vi "GDSProject_CreateClass.vi"(0 "Project Refnum In":refnum<vi>, 1 "Project Item To Create Class Below(Use MyComputer if not wired)":refnum<vi>, 2 "ClassFolder":path=path "C:/Documents and Settings/Micke/Mina dokument/LabView/8.1 Beta/Projects/ClassFiles/MyClass3.lvclass", 3 "ClassName":string, 5 "error in (no error)":errorcluster) -> (14 "Project Refnum Out":refnum<vi>, 15 "Class Refnum Out":refnum<vi>, 16 "ClassPathOut":path, 19 "error out":errorcluster)   [LabVIEW 2020]
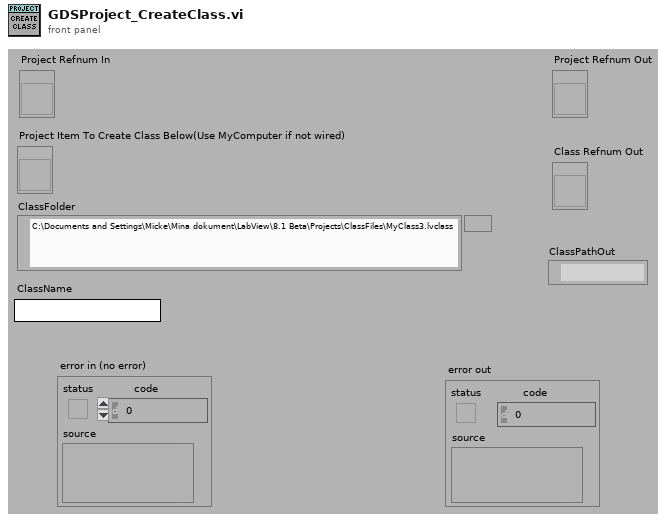
[diagram p1: front panel]
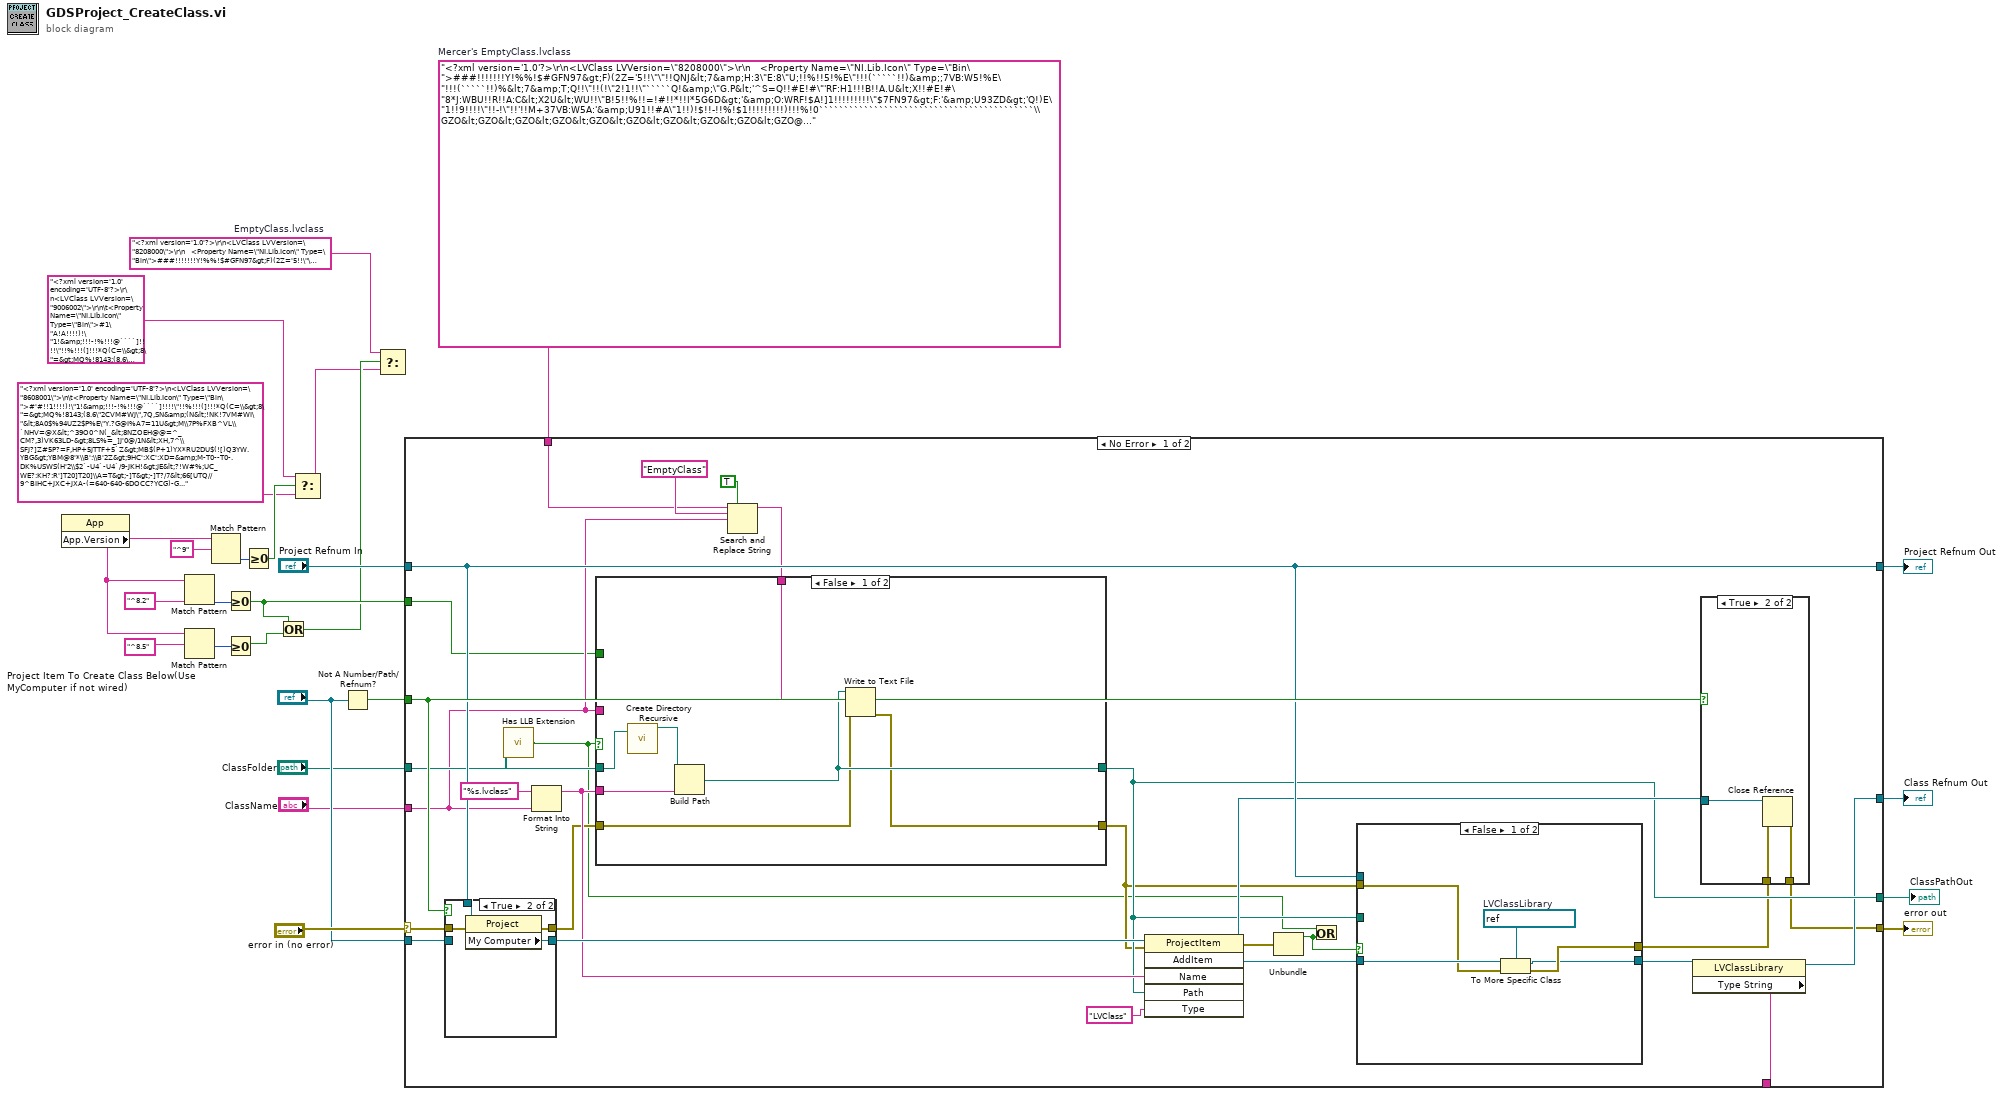
[diagram p0: block diagram]
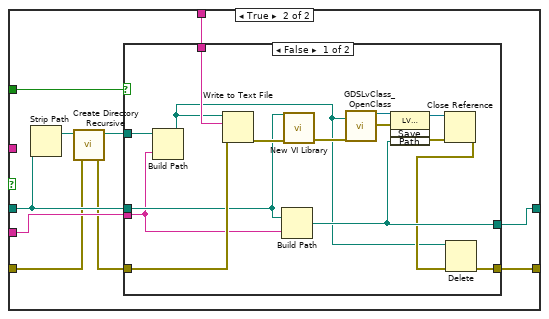
[diagram p2: hidden frame]
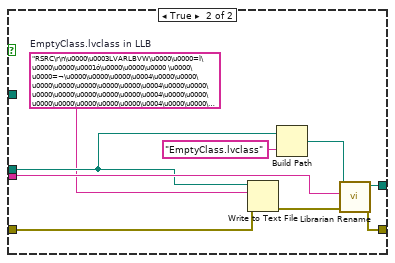
[diagram p3: hidden frame]
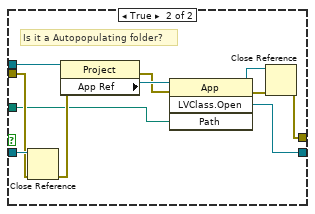
[diagram p4: hidden frame]
diagram:
  w1 = "<?xml version='1.0'?>\r\n<LVClass LVVersion=\"8208000\">\r\n   <Property Name=\"NI.Lib.Icon\" Type=\"Bin\">###!!!!!!!Y!%%!$#GFN97&gt;F)(2Z='5!!\"\"!!QNJ&lt;7&amp;H:3\"E:8\"U;!!%!!5!%E\"!!!(`````!!)&amp;;7VB:W5!%E\"!!!(`````!!)%&lt;7&amp;T;Q!!\"!!(!\"2!1!!\"`````Q!&amp;\"G.P&lt;'^S=Q!!#E!#\"'RF:H1!!!B!!A.U&lt;X!!#E!#\"8*J:WBU!!R!!A:C&lt;X2U&lt;WU!!\"B!5!!%!!=!#!!*!!I*5G6D&gt;'&amp;O:WRF!$A!]1!!!!!!!!!\"$7FN97&gt;F:'&amp;U93ZD&gt;'Q!)E\"1!!9!!!!\"!!-!\"!!'!!M+37VB:W5A:'&amp;U91!!#A\"1!!)!$!!-!!%!$1!!!!!!!!!)!!!%!0```````````````````````````````````````````\\GZO&lt;GZO&lt;GZO&lt;GZO&lt;GZO&lt;GZO&lt;GZO&lt;GZO&lt;GZO&lt;GZO@``O&lt;GZO&lt;GZO&lt;GZO&lt;GZO&lt;GZO&lt;GZO&lt;GZO&lt;GZO&lt;GZ`\\GZ``_ZO&lt;GZO&lt;GZO&lt;GZO&lt;GZO&lt;GZO&lt;GZO&lt;GZO&lt;GZO@``O&lt;H``\\GZO&lt;GZO&lt;GZO&lt;GZO&lt;GZO&lt;GZO&lt;GZO&lt;GZO&lt;GZO@_ZO@``O&lt;GZO&lt;GZO&lt;GZO&lt;GZO&lt;GZO&lt;GZO&lt;GZO&lt;GZO&lt;GZ`\\GZ``_ZO&lt;GZO&lt;GZO&lt;GZO&lt;GZO&lt;GZO&lt;GZO&lt;GZO&lt;GZO&lt;H`O&lt;H``\\GZO&lt;GZO&lt;GZO&lt;GZO&lt;GZO&lt;GZO&lt;GZO&lt;GZO&lt;GZO@_ZO@``O&lt;GZO&lt;GZO&lt;GZO&lt;GZO&lt;GZO&lt;GZO&lt;GZO&lt;GZO&lt;GZ`\\GZ``_ZO&lt;GZO&lt;GZO&lt;GZO&lt;GZO&lt;GZO&lt;GZO&lt;GZO&lt;GZO@```\\H``\\GZO&lt;GZO&lt;GZO&lt;GZO&lt;GZO&lt;GZO&lt;GZO&lt;GZO&lt;GZO&lt;GZO@```\\H`O@_Z`\\H`O@_Z`\\H`O@_Z`\\H`O@_Z`\\H`O@_Z``]!!!!!!!!!!!!!!!!!!!!!!!!!!!!!!!!!!!!!!!$``Q$``````````````Q!!!!!!!!!!!!!!!!!!!!!!!0``!0^%2%2%`U2%2%4`!!!!!!!!!!!!!!!!!!!!!!!!``]!`U2%2%4`2%2%20]!!!!!!!!!!!!!!!!!!!!!!!$``Q$`2%2%20^%2%2%`Q!!!!!!!!!!!!!!!!!!!!!!!0``!0^%2%2%`U2%2%4`!!!!!!!!!!!!!!!!!!!!!!!!``]!``````````````]!!!!!!!!!!!!!!!!!!!!!!!$``Q$`!!!!!0]!!!!!AY-!!!!!!!!!!!!!!!!!!!!!!0``!0]!!!!!`Q!!!!#$\"9/$!!!!!!!!!!!!!!!!!!!!``]!`Q!!!!$`!#-D)Y-&amp;\"17$AQ!!!!!!!!!!!!!!!!$``Q$`!!!!!0]!!!!!AQ5&amp;`Q5&amp;AY-!!!!!!!!!!!!!!0``!0````````````_$\"@```Q5&amp;\"9-D)Q!!!!!!!!!!``]!!!!!!!!!!!!!!)-&amp;\"@]&amp;\"9/$!!!!!!!!!!!!!!$``Q!!!!!!!!!!V.45AQ5&amp;\"9/$!!!!!!!!!!!!!!!!!0``!!!!!!!!!!!!!!#$\"9/$!!!!!!!!!!!!!!!!!!!!``]!!!!!!!!!!!!!!)/$!!!!!!!!!!!!!!!!!!!!!!$``Q!!!!!!!!!!!!!!!!!!!!!!!!!!!!!!!!!!!!!!!0``!!!!!!!!!!!!!!!!!!!!!!!!!!!!!!!!!!!!!!!!``]!!!!!!!!!!!!!!!!!!!!!!!!!!!!!!!!!!!!!!!$```````````````````````````````````````````]!!!#!``````````````````````````````````````````````````````````````````````````````````````````````````````````````````````````````````````````````````````````````````````````]!!!%!!0```Q$``]Q!``_:!0``:A$``T-!``]!!0`-`Q$`T-Q!`]S:!0`-:A$`T$-!`]Q!!0_:`Q$`G=Q!`ZG:!0_::A$`G4-!`ZE!!0^G`Q$`:MQ!`W;:!0^G:A$`:D-!`W9!!0]T`Q$`-]Q!`T/:!0]T:A$`-T-!`T-!!0]!`Q$`!-Q!`Q#:!0]!:A$`!$-!`Q!!!-T``Q$-`]Q!T0_:!-T`:A$-`T-!T0]!!-T-`Q$-T-Q!T-S:!-T-:A$-T$-!T-Q!!-S:`Q$-G=Q!T*G:!-S::A$-G4-!T*E!!-RG`Q$-:MQ!T';:!-RG:A$-:D-!T'9!!-QT`Q$--]Q!T$/:!-QT:A$--T-!T$-!!-Q!`Q$-!-Q!T!#:!-Q!:A$-!$-!T!!!!*H``Q#:`]Q!G@_:!*H`:A#:`T-!G@]!!*H-`Q#:T-Q!G=S:!*H-:A#:T$-!G=Q!!*G:`Q#:G=Q!G:G:!*G::A#:G4-!G:E!!*FG`Q#::MQ!G7;:!*FG:A#::D-!G79!!*ET`Q#:-]Q!G4/:!*ET:A#:-T-!G4-!!*E!`Q#:!-Q!G1#:!*E!:A#:!$-!G1!!!'&lt;``Q\"G`]Q!:P_:!'&lt;`:A\"G`T-!:P]!!'&lt;-`Q\"GT-Q!:MS:!'&lt;-:A\"GT$-!:MQ!!';:`Q\"GG=Q!:JG:!';::A\"GG4-!:JE!!':G`Q\"G:MQ!:G;:!':G:A\"G:D-!:G9!!'9T`Q\"G-]Q!:D/:!'9T:A\"G-T-!:D-!!'9!`Q\"G!-Q!:A#:!'9!:A\"G!$-!:A!!!$0``Q!T`]Q!-`_:!$0`:A!T`T-!-`]!!$0-`Q!TT-Q!-]S:!$0-:A!TT$-!-]Q!!$/:`Q!TG=Q!-ZG:!$/::A!TG4-!-ZE!!$.G`Q!T:MQ!-W;:!$.G:A!T:D-!-W9!!$-T`Q!T-]Q!-T/:!$-T:A!T-T-!-T-!!$-!`Q!T!-Q!-Q#:!$-!:A!T!$-!-Q!!!!$``Q!!`]Q!!0_:!!$`:A!!`T-!!0]!!!$-`Q!!T-Q!!-S:!!$-:A!!T$-!!-Q!!!#:`Q!!G=Q!!*G:!!#::A!!G4-!!*E!!!\"G`Q!!:MQ!!';:!!\"G:A!!:D-!!'9!!!!T`Q!!-]Q!!$/:!!!T:A!!-T-!!$-!!!!!`Q!!!-Q!!!#:!!!!:A!!!$-!\\A!!!.U!!!#\\!!!!KA!!!)A!!!\"X!!!!61!!!%1!!!!C!!!!%1!!!!$O!!!!X1!!!,M!!!#K!!!!C!!!!(=!!!\"6!!!!2!!!!#)!!!!2!!!!!/Y!!!$&gt;!!!!OQ!!!+I!!!#)!!!!&gt;Q!!!&amp;5!!!\"%!!!!)A!!!\"%!\\O\\O!.X&gt;X1#\\O\\M!KKKK!)C)C!\"X&gt;X=!6666!%2%2!!C)C)!%2%2!!!!!!!!!!!!)!!A!!!!!!!!!!%!!!#!`````Y!!!!'!!!!*A!!!'9!!!!G!!!!*A!!!#9!!!!G!!!!*A!!!(9!!!!(`````A!!!!&lt;`Y!!'TG!!\"L7A!!;VI!!'TG!!\"P`!!!;%-!!'B?Q!\"I8D!!;%*)!'`[ZY\"A!EA!9\"YQ!'!?Q!\"A!Q!!9!!!!'!!!!\"A!!!!@````]!!!#!``````````````````````````````````````````````````````````````````````````````````````````````````````````````````````````````````````````````````````````````````````````]!!!!#!0```Q!!!!!!!!!!!#!!)!!!!!!</Property>\r\n   <Property Name=\"NI.Lib.Version\" Type=\"Str\">1.0.0.0</Property>\r\n   <Property Name=\"NI.LVClass.ClassNameVisibleInProbe\" Type=\"Bool\">true</Property>\r\n   <Property Name=\"NI.LVClass.FlattenedPrivateDataCTL\" Type=\"Bin\">###!!!!!!!)!\"!!&amp;!!Q!1!!\"`````Q!!!!%!!1!!%VB35V*$$1I!!UR71U.-1F:8!!!0_!!!!W!!!!!A!!!0W!!!!\"=!!!!\"%E6N=(2Z1WRB=X-O&lt;(:D&lt;'&amp;T=Q!!!!\"Q##'!!A!Q!!!)!!!!!!!!\"!!$!$Q!P!!@1!!#!!!!!!%!!1!'`````Q!!!!!!!!!!!!!!!!!!!!!!!!!!!!!!!!!!!!!!!!!'!!!!%!!!!!!!!!!!!!!!!!!!!!!!!!!!V\"W-W9]!MA4JA!G9\\0B#@A!!!']!!5R71U-B27VQ&gt;(F$&lt;'&amp;T=SZM&gt;G.M98.T/E6N=(2Z1WRB=X-O9X2M!!!!!!!\"!!*735R#!!!!!2*&amp;&lt;8\"U?5.M98.T,GRW9WRB=X-!5&amp;2)-!!!!\"E!!1!$!!!327VQ&gt;(F$&lt;'&amp;T=SZM&gt;G.M98.T!!-!!!!!7A!!!!%!5A$RQOG`-1!!!!)327VQ&gt;(F$&lt;'&amp;T=SZM&gt;G.M98.T$E6N=(2Z1WRB=X-O9X2M!$J!5!!!(5.M&gt;8.U:8)A&lt;W9A9WRB=X-A=(*J&gt;G&amp;U:3\"E982B!!%!!!!!!!!\";!!!!\"I!#A\"D!!!\"?!!%!!1!!Q!+!'1!!!!Q!!%!#!\"A!!!!$!!+!&amp;!!!A!#!!-!#A\"D!!!!-!!\"!!B!\"Q.G&lt;'=!#%!(!W^3&gt;!!)1!=$:7^G!\"\"!5!!$!!9!\"Q!)!X6E:A!E1&amp;!!!\"V$&lt;(6T&gt;'6S)'^G)'.M98.T)(\"S;8:B&gt;'5A:'&amp;U91!+1&amp;!!!!.E:G1!#E\"1!!!$&gt;(BE!!J!5!!!!W^M:!!+1&amp;!!!!.F?(1!%A\"1!!9!#1!+!!M!$!!.!!Y!#A\"D!!!!*!!\"!!9!AQ!+!!I!9Q!!!!A!\"!!+!'-!!!!!!!1!\"!!#!!1!!1!)!'!!!!!%!$Y!5!!=!\"1!&amp;!!6!\"5!&amp;1!6!!%!!1!\"!\"5!&amp;1!6!\"5!!1!\"!!%!!1!6!\"5!&amp;1!6!\"5!&amp;1!6!\"5!&amp;A!7!\"9!#A\"E!!!!!1!8!!1!!!!+!!!1!!!%%!%!\"2!!!!]1\"!!1%!!!%2!!!\")1!!!4%!!!'$!!!\"E1!!!!!%!!!!%)?*RD9-!*'\"E9G$9!;1[9Q(]AA)IX!'E7X&amp;L*\"V!\\-.DYR&amp;!\")V#?K14)9%;)A&gt;Q,&gt;D-=M+(J!A$&amp;D2/W!!!!-!!\"6EF%5S&amp;&amp;&lt;8\"U?5.M98.T,GRW9WRB=X-[27VQ&gt;(F$&lt;'&amp;T=SZD&gt;'Q!!!!!!!!!!Q!!!*Y!!!$E?*T,9W\"AS$3W-&amp;P&amp;A!$*_3GJ)0I#%(?_W'=)IAJYDDPI#!*:!;(&gt;LAT`\"8J46$BM19J+W8?!K--4`D_9-'&amp;#@&amp;R5:(4MY1GBX4EK(-'\"17(B/RC\"MJD#X;5-/]*\"\"LNJ\\&amp;!!UQY\\]M#U3Q:)2_A,E+EA7W\"[:Q(Z:Y&amp;3).H`1-$)Q-+AT&amp;$$U-,1A_2W:X]86S1OW!]!1%1X?!!!!!!!#QAAA!!!!!-Y,D)!!!!!!)$`````A!!!!9!!!!'!!!!\"A!Q!!9!T!!'!Q-!\"AQ!Q!91!#!''!!A\"B9!Y!92A[!'%'VA\"B!;I!91&amp;7!'%\"KA\"B!69!91'K!'%\"6]\"AQ;PQ9$&amp;8Q'!.PY\"A!`Y#9!\"Y\"G!!!!*A!!!#9!!!!G!!!!*A!!!#9!!!\"W!!!!\"`````Q!!\"!$```````````````````````````````````````````]!!!!!!!!!!!!!!!!!!!!!!!!!!!!!!!!!!!!!!!$``Q!!!!!!!!!!!!!!!!!!!!!!!!!!!!!!!!!!!!!!!0``!!!!!!!!!!!!!!!!!!!!!!!!!!!!!!!!!!!!!!!!``]!!!!!!!!!!!!!!*35!!!!!!!!!!!!!!!!!!!!!!$``Q!!!!!!!!!!!*3GI+;GF!!!!!!!!!!!!!!!!!!!!0``!!!!!!!!!*3GI*K;GJKGJJ1!!!!!!!!!!!!!!!!!``]!!!!!!*3GI*K;GJK;GJK;JK;5!!!!!!!!!!!!!!$``Q!!!!#GI*K;GJK;GJK;GJK;GK;G!!!!!!!!!!!!!0``!!!!!+#AGJK;GJK;GJK;GJK;L+9!!!!!!!!!!!!!``]!!!!!I+;GI*K;GJK;GJK;L+SMI!!!!!!!!!!!!!$``Q!!!!#AJK;GJK#;GJK;L+SML+SA!!!!!!!!!!!!!0``!!!!!+#GJK;GJK;AJKSML+SML+!!!!!!!!!!!!!!``]!!!!!I+;GJK;GJK;ML+SML+SMI!!!!!!!!!!!!!$``Q!!!!#AJK;GJK;GJKSML+SML+SA!!!!!!!!!!!!!0``!!!!!+#GJK;GJK;GL+SML+SML+!!!!!!!!!!!!!!``]!!!!!I+;GJK;GJK;ML+SML+SMI!!!!!!!!!!!!!$``Q!!!!#AJK;GJK;GJKSML+SML+SA!!!!!!!!!!!!!0``!!!!!+;GJK;GJK;GL+SML+SMJK9L+SM!!!!!!!!!``]!!!!!!+#AJK;GJK;ML+SMJK;A+SML+SML!!!!!!$``Q!!!!!!!!#AJK;GJKSMJK;A+SML+SML!!!!!!!!!0``!!!!!!!!!!!!I+;GJK;;+SML+SML+Q!!!!!!!!!!``]!!!!!!!!!!!!!!+#;+SML+SML+Q!!!!!!!!$`!!$``Q!!!!!!!!!!!!!!!!!!+SML+Q!!!!!!!!!!``]!!0``!!!!!!!!!!!!!!!!!!!!!!!!!!!!!!!!!!!!`Q!!``]!!!!!!!!!!!!!!!!!!!!!!!!!!!!!!!!!!!$`!!$``Q!!!!!!!!!!!!!!!!!!!!!!!!!!!!!!!!!!!0]!!0``!!!!!!!!!!!!!!!!!!!!!!!!!!!!!!!!!!!!`Q!!``]!!!!!!!!!!!!!!!!!!!!!!!!!!!!!!!!!!!$`!!$``Q!!!!!!!!!!!!!!!!!!!!!!!!!!!!!!!!!!````!0``!!!!!!!!!!!!!!!!!!!!!!!!!!!!!!!!!!!!!!!!````````````````````````````````````````````!!!!4!!!!!%!2!$RQOG`-1!!!!)(1WRB=X-A-1N$&lt;'&amp;T=S!R,G.U&lt;!!Q1&amp;!!!\"V$&lt;(6T&gt;'6S)'^G)'.M98.T)(\"S;8:B&gt;'5A:'&amp;U91!\"!!!!!!!Q!!!!!1!E1&amp;!!!\"V$&lt;(6T&gt;'6S)'^G)'.M98.T)(\"S;8:B&gt;'5A:'&amp;U91!$!!!!!!!!!!!!-!!\"2F\")5#&amp;&amp;&lt;8\"U?5.M98.T,GRW9WRB=X-[27VQ&gt;(F$&lt;'&amp;T=SZD&gt;'Q!!!!!!!!!!Q!!!&amp;!!!!!!!!!%\"!!!!!!!&amp;A!&amp;!#-!(A!!!\"9!!!!'!!!!)Q!!!\"Y!!!!!!1!!!!!!!!!!!!!!!!!!!!!!!!!!!!!!!!!!#A!!!!!!!!!%5'&amp;O:1!!!'E!!!!!!!!%\"!!!!!!!!Q!\"!\"!!C1!!!!-!!!!#!!!!%!!!!)E!!!!!!1!!!!!!!!!!!!!!!!!!!!!!!!!!!!!!!!!!#A!!!!!!!!!&gt;1WRV=X2F=C\"P:C\"D&lt;'&amp;T=S\"Q=GFW982F)'2B&gt;'%!!!!!!!\"1!!!!!!!!\"!1!!!!!!!%!!1!/!\"I!!!!\"!!!!!A!!!!Y!!!!;!!!!!!%!!!!!!!!!!!!!!!!!!!!!!!!!!!!!!!!!!!I!!!!!!!!!\"&amp;\"B&lt;G5!!!*X!!!&amp;&amp;HC=H:1`;\".2(-&gt;`\\Z,I3T$U*5WVQ5CCP,2&amp;UM7`.@CHVN?B5AI3#QY\"/RTI&amp;IJ5H&gt;LFFB1#!3'$U,&amp;:(4)I4E8C&gt;)O41TO%TCY/&amp;O8M8@S^/^`F'CY/8MDFXLXX_8X@\\`O_\"##7:J/;!ZMW%(;%$]MW*.AC0GT:-#%?J0=_*SH)KQ#&amp;9OYU`UC%G&gt;ZD3_1X!FHCE\"_:0,%\"?!(Y2?B?]B@4,&amp;WCCWR(=QD/H[5\\&lt;&amp;5SG3S/ZOEK/]#*H!VH^(W3@'3]\"Q,%_#,:\\F/P\"F[J&amp;5]GYE!;+1O!68\"L&amp;2MOO^6A5/?+W#&gt;%F?E@^Y_(SU\"]B2XC\\SGX8-+'[VD/K\"'=.W&lt;EH@=9@Z@D^6BXVC0(Y,ROHEM^:!XC;%^Y`C&gt;N&amp;'=VGH5,R'WY9;(7$(1[(&gt;[&lt;2F45Y:0(6P'T,MQ,GQI&amp;WBBQ.SX1&amp;$@F3MZ*L)LA/F2(9H-72)S;R\"2==O'%\"[/CK\\HFQ3,PP!H3NSS))NVKN23.['P6;F8KMB=+N?&gt;^^,E.:1NCP,?!;`P@U&amp;H]YNE?9L@@*4Y\"562?U]WJ6#;Y\\Y.C78-.DSL$&lt;Y=:(B&gt;V\"L+/*A]+NK8D#S==DQS;O#-&gt;LU'\\X=9G]#[&lt;E\"6/\\%39W;OB\"N[6PP]VU.0XU21/.U\"(&gt;.SX4Q^[=!`.&amp;\\]?0`.]5-'30KDB\"GQ&lt;JL&lt;'IL23H)ZQU3_7)])EO'9Y?'0`&amp;&lt;TII\"%W+HCE35JE6ZD*F[%'J%+$2UI)XC@.E6D[(]&amp;$P3&lt;#5P.6?0$'P?!&amp;[%$Q*-\\.%&lt;H,_,E,_KW/$.R&gt;\\W,O[,7BX%%!U@%)A\"ZVP`JPOMP_I`?(Q^`GD1`OU(&amp;&amp;*P]!ITNFNQ!!!!!)!!!!)!!!\"5A!!!!Q!!&amp;#2%B1)56N=(2Z1WRB=X-O&lt;(:D&lt;'&amp;T=TJ&amp;&lt;8\"U?5.M98.T,G.U&lt;!!!!!!!!!!$!!!!@!!!!*6YH'.A9*AI)-(UD[(O,Q/4Q&amp;=A1`IP!\\/A(_.P\"A:/0Y($1*J21*,Z(Y0M8Q&lt;W8QQ-ANJA'?UDOBQ-5+$+RKBCR?2SGIG\"1Z,DM#!(7!&amp;(CQ&lt;$````69I9Q2*@DVS$KT`C!W?W8!#2+L0E7X;!O@^!*)=%!&amp;UH)5E!!!!)!!!!\"Q!!!1!!!!$`!!!!\"!!!!\"J-6E.M98.T5(*J&gt;G&amp;U:52B&gt;'&amp;597*0=G2F=AABA!)!!!!#!!1!\"Q!-!%!!!@````]!!!!\"!!%!!!!!!!!!!!!!!\"N-6E.M98.T5(*J&gt;G&amp;U:52B&gt;'&amp;5;7VF=X2B&lt;8!))9!#!!!!!1!%!!=!!1!!QOG`-1!!!!!!!!!;4&amp;:$&lt;'&amp;T=V\"S;8:B&gt;'6%982B6(FQ:52F=W-))9!#!!!!!1!)!$$`````!!%!!!!!!!Y!!!!\"!!9!5!!!!!%!!!!!!!!!!!!?4&amp;:$&lt;'&amp;T=V\"S;8:B&gt;'6%982B2':M&gt;%2B&gt;'&amp;4;8JF##'!!A!!!!%!\"!!$!!%!!!!!!!!!!!!!!!!!!!1!!!\"!!!!!+!!!!!)!!!1!!!!!!1!!!!!!!!!!!!!!!!!!!!!!!!!!!!!!!!!!!!!!!!$`!!%!!A!$!!Y!!!$I!!Y%!!!!!!Y!ZQ$7!!!!\\Q!/\"!!!!!!/!/=!VA!!!09!$A1!!!!!$A$H!.9!!!!!!!!!!!!!!!!!!!!!!!!!!!!!!!!!!!!!!!!!!!!!!!!!!!!!!!!!!!!!!!!!!!!!!!!!!!!!!!!!!!!!!!!!!!!!!!!!!!!!!!!!!!!!!!!!!!!!!!!!!!!!!!!!!!!!!!!!!!!!!!!!!!!!!!!!!!!!!!!!!!!!!!!!!!!!!!!!!!!!!!!!!!!!!!!!!!!!!!!!!!!!!!!!!!!!!!!!`1!.B!#!!!!.!.!!O1:597BP&lt;7%'6'&amp;I&lt;WVB\"F2B;'^N91%R!&amp;*45E-.#A!$4&amp;:$1UR#6F=!!!`Y!!!$9!!!!#!!!!`9!!!!!!!!!!!!!!!A!!!!.!!!!!!!!!!84%F#4A!!!!!!!!%E4&amp;:45A!!!!!!!!%Y4%FW;1!!!!!!!!&amp;-1U^/5!!!!!!!!!&amp;A6%UY-!!!!!!!!!&amp;U2%:%5Q!!!!!!!!')4%FE=Q!!!!!!!!'=6EF$2!!!!!!!!!'Q&gt;G6S=Q!!!!!!!!(%35.04A!!!!!!!!(9;7.M/!!!!!!!!!(M1V\"$-A!!!!!!!!)!2&amp;2)5!!!!!!!!!)54%FG=!!!!!!!!!)I6&amp;*F9Q!!!!)!!!)]2F\")9A!!!!!!!!*Y2F\"421!!!!!!!!+-4%FC:!!!!!!!!!+A1E2)9A!!!!!!!!+U1E2421!!!!!!!!,)6EF55Q!!!!!!!!,=466*2!!!!!!!!!,Q3%F46!!!!!!!!!-%2F2\"1A!!!!!!!!-9!!!!!0````]!!!!!!!!!!$D'MAI!!!!!`````Q!!!!!!!!!=,-;S#A!!!!$`````!!!!!!!!!*!ARL)+!!!!!0````]!!!!!!!!\"\"\"4'MAI!!!!!`````Q!!!!!!!!&amp;E#-;S#A!!!!$`````!!!!!!!!!N$]R&lt;)+!!!!!0````]!!!!!!!!$&amp;0$&amp;MAI!!!!!`````Q!!!!!!!!.)Z-7S#A!!!!4`````!!!!!!!!!_T9R&lt;)+!!!!!0````]!!!!!!!!$`-T&amp;MAI!!!!!`````Q!!!!!!!!3!Q-7S#A!!!!$`````!!!!!!!!#)3UR&lt;)+!!!!!0````]!!!!!!!!)V+D&amp;MAI!!!!!`````Q!!!!!!!!E)H-7S#A!!!!,`````!!!!!!!!#4S1R&lt;)+!!!!!`````]!!!!!!!!*E)4&amp;MAI!!!!%`````Q!!!!!!!!I!?-7S#A!!!!$`````!!!!!!!!#F2MR&lt;)+!!!!!0````]!!!!!!!!-U'$&amp;MAI!!!!!`````Q!!!!!!!!T=6-7S#A!!!!$`````!!!!!!!!$2\")R&lt;)+!!!!!0````]!!!!!!!!.E$T&amp;MAI!!!!!`````Q!!!!!!!!W=--7S#A!!!!$`````!!!!!!!!$K!ER&lt;)+!!!!!0````]!!!!!!!!/K\"D&amp;MAI!!!#!`````Q!!!!!!!!\\5$-7S#A!!!!!</Property>\r\n   <Item Name=\"EmptyClass.ctl\" Type=\"Class Private Data\" URL=\"EmptyClass.lvclass/EmptyClass.ctl\">\r\n      <Property Name=\"NI.LibItem.Scope\" Type=\"Int\">2</Property>\r\n   </Item>\r\n</LVClass>\r\n"  # Mercer's EmptyClass.lvclass
  w9 = "<?xml version='1.0'?>\r\n<LVClass LVVersion=\"8208000\">\r\n   <Property Name=\"NI.Lib.Icon\" Type=\"Bin\">###!!!!!!!Y!%%!$#GFN97&gt;F)(2Z='5!!\"\"!!QNJ&lt;7&amp;H:3\"E:8\"U;!!%!!5!%E\"!!!(`````!!)&amp;;7VB:W5!%E\"!!!(`````!!)%&lt;7&amp;T;Q!!\"!!(!\"2!1!!\"`````Q!&amp;\"G.P&lt;'^S=Q!!#E!#\"'RF:H1!!!B!!A.U&lt;X!!#E!#\"8*J:WBU!!R!!A:C&lt;X2U&lt;WU!!\"B!5!!%!!=!#!!*!!I*5G6D&gt;'&amp;O:WRF!$A!]1!!!!!!!!!\"$7FN97&gt;F:'&amp;U93ZD&gt;'Q!)E\"1!!9!!!!\"!!-!\"!!'!!M+37VB:W5A:'&amp;U91!!#A\"1!!)!$!!-!!%!$1!!!!!!!!!)!!!%!0```````````````````````````````````````````\\GZO&lt;GZO&lt;GZO&lt;GZO&lt;GZO&lt;GZO&lt;GZO&lt;GZO&lt;GZO&lt;GZO@``O&lt;GZO&lt;GZO&lt;GZO&lt;GZO&lt;GZO&lt;GZO&lt;GZO&lt;GZO&lt;GZ`\\GZ``_ZO&lt;GZO&lt;GZO&lt;GZO&lt;GZO&lt;GZO&lt;GZO&lt;GZO&lt;GZO@``O&lt;H``\\GZO&lt;GZO&lt;GZO&lt;GZO&lt;GZO&lt;GZO&lt;GZO&lt;GZO&lt;GZO@_ZO@``O&lt;GZO&lt;GZO&lt;GZO&lt;GZO&lt;GZO&lt;GZO&lt;GZO&lt;GZO&lt;GZ`\\GZ``_ZO&lt;GZO&lt;GZO&lt;GZO&lt;GZO&lt;GZO&lt;GZO&lt;GZO&lt;GZO&lt;H`O&lt;H``\\GZO&lt;GZO&lt;GZO&lt;GZO&lt;GZO&lt;GZO&lt;GZO&lt;GZO&lt;GZO@_ZO@``O&lt;GZO&lt;GZO&lt;GZO&lt;GZO&lt;GZO&lt;GZO&lt;GZO&lt;GZO&lt;GZ`\\GZ``_ZO&lt;GZO&lt;GZO&lt;GZO&lt;GZO&lt;GZO&lt;GZO&lt;GZO&lt;GZO@```\\H``\\GZO&lt;GZO&lt;GZO&lt;GZO&lt;GZO&lt;GZO&lt;GZO&lt;GZO&lt;GZO&lt;GZO@```\\H`O@_Z`\\H`O@_Z`\\H`O@_Z`\\H`O@_Z`\\H`O@_Z``]!!!!!!!!!!!!!!!!!!!!!!!!!!!!!!!!!!!!!!!$``Q$``````````````Q!!!!!!!!!!!!!!!!!!!!!!!0``!0^%2%2%`U2%2%4`!!!!!!!!!!!!!!!!!!!!!!!!``]!`U2%2%4`2%2%20]!!!!!!!!!!!!!!!!!!!!!!!$``Q$`2%2%20^%2%2%`Q!!!!!!!!!!!!!!!!!!!!!!!0``!0^%2%2%`U2%2%4`!!!!!!!!!!!!!!!!!!!!!!!!``]!``````````````]!!!!!!!!!!!!!!!!!!!!!!!$``Q$`!!!!!0]!!!!!AY-!!!!!!!!!!!!!!!!!!!!!!0``!0]!!!!!`Q!!!!#$\"9/$!!!!!!!!!!!!!!!!!!!!``]!`Q!!!!$`!#-D)Y-&amp;\"17$AQ!!!!!!!!!!!!!!!!$``Q$`!!!!!0]!!!!!AQ5&amp;`Q5&amp;AY-!!!!!!!!!!!!!!0``!0````````````_$\"@```Q5&amp;\"9-D)Q!!!!!!!!!!``]!!!!!!!!!!!!!!)-&amp;\"@]&amp;\"9/$!!!!!!!!!!!!!!$``Q!!!!!!!!!!V.45AQ5&amp;\"9/$!!!!!!!!!!!!!!!!!0``!!!!!!!!!!!!!!#$\"9/$!!!!!!!!!!!!!!!!!!!!``]!!!!!!!!!!!!!!)/$!!!!!!!!!!!!!!!!!!!!!!$``Q!!!!!!!!!!!!!!!!!!!!!!!!!!!!!!!!!!!!!!!0``!!!!!!!!!!!!!!!!!!!!!!!!!!!!!!!!!!!!!!!!``]!!!!!!!!!!!!!!!!!!!!!!!!!!!!!!!!!!!!!!!$```````````````````````````````````````````]!!!#!``````````````````````````````````````````````````````````````````````````````````````````````````````````````````````````````````````````````````````````````````````````]!!!%!!0```Q$``]Q!``_:!0``:A$``T-!``]!!0`-`Q$`T-Q!`]S:!0`-:A$`T$-!`]Q!!0_:`Q$`G=Q!`ZG:!0_::A$`G4-!`ZE!!0^G`Q$`:MQ!`W;:!0^G:A$`:D-!`W9!!0]T`Q$`-]Q!`T/:!0]T:A$`-T-!`T-!!0]!`Q$`!-Q!`Q#:!0]!:A$`!$-!`Q!!!-T``Q$-`]Q!T0_:!-T`:A$-`T-!T0]!!-T-`Q$-T-Q!T-S:!-T-:A$-T$-!T-Q!!-S:`Q$-G=Q!T*G:!-S::A$-G4-!T*E!!-RG`Q$-:MQ!T';:!-RG:A$-:D-!T'9!!-QT`Q$--]Q!T$/:!-QT:A$--T-!T$-!!-Q!`Q$-!-Q!T!#:!-Q!:A$-!$-!T!!!!*H``Q#:`]Q!G@_:!*H`:A#:`T-!G@]!!*H-`Q#:T-Q!G=S:!*H-:A#:T$-!G=Q!!*G:`Q#:G=Q!G:G:!*G::A#:G4-!G:E!!*FG`Q#::MQ!G7;:!*FG:A#::D-!G79!!*ET`Q#:-]Q!G4/:!*ET:A#:-T-!G4-!!*E!`Q#:!-Q!G1#:!*E!:A#:!$-!G1!!!'&lt;``Q\"G`]Q!:P_:!'&lt;`:A\"G`T-!:P]!!'&lt;-`Q\"GT-Q!:MS:!'&lt;-:A\"GT$-!:MQ!!';:`Q\"GG=Q!:JG:!';::A\"GG4-!:JE!!':G`Q\"G:MQ!:G;:!':G:A\"G:D-!:G9!!'9T`Q\"G-]Q!:D/:!'9T:A\"G-T-!:D-!!'9!`Q\"G!-Q!:A#:!'9!:A\"G!$-!:A!!!$0``Q!T`]Q!-`_:!$0`:A!T`T-!-`]!!$0-`Q!TT-Q!-]S:!$0-:A!TT$-!-]Q!!$/:`Q!TG=Q!-ZG:!$/::A!TG4-!-ZE!!$.G`Q!T:MQ!-W;:!$.G:A!T:D-!-W9!!$-T`Q!T-]Q!-T/:!$-T:A!T-T-!-T-!!$-!`Q!T!-Q!-Q#:!$-!:A!T!$-!-Q!!!!$``Q!!`]Q!!0_:!!$`:A!!`T-!!0]!!!$-`Q!!T-Q!!-S:!!$-:A!!T$-!!-Q!!!#:`Q!!G=Q!!*G:!!#::A!!G4-!!*E!!!\"G`Q!!:MQ!!';:!!\"G:A!!:D-!!'9!!!!T`Q!!-]Q!!$/:!!!T:A!!-T-!!$-!!!!!`Q!!!-Q!!!#:!!!!:A!!!$-!\\A!!!.U!!!#\\!!!!KA!!!)A!!!\"X!!!!61!!!%1!!!!C!!!!%1!!!!$O!!!!X1!!!,M!!!#K!!!!C!!!!(=!!!\"6!!!!2!!!!#)!!!!2!!!!!/Y!!!$&gt;!!!!OQ!!!+I!!!#)!!!!&gt;Q!!!&amp;5!!!\"%!!!!)A!!!\"%!\\O\\O!.X&gt;X1#\\O\\M!KKKK!)C)C!\"X&gt;X=!6666!%2%2!!C)C)!%2%2!!!!!!!!!!!!)!!A!!!!!!!!!!%!!!#!`````Y!!!!'!!!!*A!!!'9!!!!G!!!!*A!!!#9!!!!G!!!!*A!!!(9!!!!(`````A!!!!&lt;`Y!!'TG!!\"L7A!!;VI!!'TG!!\"P`!!!;%-!!'B?Q!\"I8D!!;%*)!'`[ZY\"A!EA!9\"YQ!'!?Q!\"A!Q!!9!!!!'!!!!\"A!!!!@````]!!!#!``````````````````````````````````````````````````````````````````````````````````````````````````````````````````````````````````````````````````````````````````````````]!!!!#!0```Q!!!!!!!!!!!#!!)!!!!!!</Property>\r\n   <Property Name=\"NI.Lib.Version\" Type=\"Str\">1.0.0.0</Property>\r\n   <Property Name=\"NI.LVClass.ClassNameVisibleInProbe\" Type=\"Bool\">true</Property>\r\n   <Property Name=\"NI.LVClass.FlattenedPrivateDataCTL\" Type=\"Bin\">###!!!!!!!)!\"!!&amp;!!Q!1!!\"`````Q!!!!%!!1!!%VB35V*$$1I!!UR71U.-1F:8!!!0_!!!!W!!!!!A!!!0W!!!!\"=!!!!\"%E6N=(2Z1WRB=X-O&lt;(:D&lt;'&amp;T=Q!!!!\"Q##'!!A!Q!!!)!!!!!!!!\"!!$!$Q!P!!@1!!#!!!!!!%!!1!'`````Q!!!!!!!!!!!!!!!!!!!!!!!!!!!!!!!!!!!!!!!!!'!!!!%!!!!!!!!!!!!!!!!!!!!!!!!!!!V\"W-W9]!MA4JA!G9\\0B#@A!!!']!!5R71U-B27VQ&gt;(F$&lt;'&amp;T=SZM&gt;G.M98.T/E6N=(2Z1WRB=X-O9X2M!!!!!!!\"!!*735R#!!!!!2*&amp;&lt;8\"U?5.M98.T,GRW9WRB=X-!5&amp;2)-!!!!\"E!!1!$!!!327VQ&gt;(F$&lt;'&amp;T=SZM&gt;G.M98.T!!-!!!!!7A!!!!%!5A$RQOG`-1!!!!)327VQ&gt;(F$&lt;'&amp;T=SZM&gt;G.M98.T$E6N=(2Z1WRB=X-O9X2M!$J!5!!!(5.M&gt;8.U:8)A&lt;W9A9WRB=X-A=(*J&gt;G&amp;U:3\"E982B!!%!!!!!!!!\";!!!!\"I!#A\"D!!!\"?!!%!!1!!Q!+!'1!!!!Q!!%!#!\"A!!!!$!!+!&amp;!!!A!#!!-!#A\"D!!!!-!!\"!!B!\"Q.G&lt;'=!#%!(!W^3&gt;!!)1!=$:7^G!\"\"!5!!$!!9!\"Q!)!X6E:A!E1&amp;!!!\"V$&lt;(6T&gt;'6S)'^G)'.M98.T)(\"S;8:B&gt;'5A:'&amp;U91!+1&amp;!!!!.E:G1!#E\"1!!!$&gt;(BE!!J!5!!!!W^M:!!+1&amp;!!!!.F?(1!%A\"1!!9!#1!+!!M!$!!.!!Y!#A\"D!!!!*!!\"!!9!AQ!+!!I!9Q!!!!A!\"!!+!'-!!!!!!!1!\"!!#!!1!!1!)!'!!!!!%!$Y!5!!=!\"1!&amp;!!6!\"5!&amp;1!6!!%!!1!\"!\"5!&amp;1!6!\"5!!1!\"!!%!!1!6!\"5!&amp;1!6!\"5!&amp;1!6!\"5!&amp;A!7!\"9!#A\"E!!!!!1!8!!1!!!!+!!!1!!!%%!%!\"2!!!!]1\"!!1%!!!%2!!!\")1!!!4%!!!'$!!!\"E1!!!!!%!!!!%)?*RD9-!*'\"E9G$9!;1[9Q(]AA)IX!'E7X&amp;L*\"V!\\-.DYR&amp;!\")V#?K14)9%;)A&gt;Q,&gt;D-=M+(J!A$&amp;D2/W!!!!-!!\"6EF%5S&amp;&amp;&lt;8\"U?5.M98.T,GRW9WRB=X-[27VQ&gt;(F$&lt;'&amp;T=SZD&gt;'Q!!!!!!!!!!Q!!!*Y!!!$E?*T,9W\"AS$3W-&amp;P&amp;A!$*_3GJ)0I#%(?_W'=)IAJYDDPI#!*:!;(&gt;LAT`\"8J46$BM19J+W8?!K--4`D_9-'&amp;#@&amp;R5:(4MY1GBX4EK(-'\"17(B/RC\"MJD#X;5-/]*\"\"LNJ\\&amp;!!UQY\\]M#U3Q:)2_A,E+EA7W\"[:Q(Z:Y&amp;3).H`1-$)Q-+AT&amp;$$U-,1A_2W:X]86S1OW!]!1%1X?!!!!!!!#QAAA!!!!!-Y,D)!!!!!!)$`````A!!!!9!!!!'!!!!\"A!Q!!9!T!!'!Q-!\"AQ!Q!91!#!''!!A\"B9!Y!92A[!'%'VA\"B!;I!91&amp;7!'%\"KA\"B!69!91'K!'%\"6]\"AQ;PQ9$&amp;8Q'!.PY\"A!`Y#9!\"Y\"G!!!!*A!!!#9!!!!G!!!!*A!!!#9!!!\"W!!!!\"`````Q!!\"!$```````````````````````````````````````````]!!!!!!!!!!!!!!!!!!!!!!!!!!!!!!!!!!!!!!!$``Q!!!!!!!!!!!!!!!!!!!!!!!!!!!!!!!!!!!!!!!0``!!!!!!!!!!!!!!!!!!!!!!!!!!!!!!!!!!!!!!!!``]!!!!!!!!!!!!!!*35!!!!!!!!!!!!!!!!!!!!!!$``Q!!!!!!!!!!!*3GI+;GF!!!!!!!!!!!!!!!!!!!!0``!!!!!!!!!*3GI*K;GJKGJJ1!!!!!!!!!!!!!!!!!``]!!!!!!*3GI*K;GJK;GJK;JK;5!!!!!!!!!!!!!!$``Q!!!!#GI*K;GJK;GJK;GJK;GK;G!!!!!!!!!!!!!0``!!!!!+#AGJK;GJK;GJK;GJK;L+9!!!!!!!!!!!!!``]!!!!!I+;GI*K;GJK;GJK;L+SMI!!!!!!!!!!!!!$``Q!!!!#AJK;GJK#;GJK;L+SML+SA!!!!!!!!!!!!!0``!!!!!+#GJK;GJK;AJKSML+SML+!!!!!!!!!!!!!!``]!!!!!I+;GJK;GJK;ML+SML+SMI!!!!!!!!!!!!!$``Q!!!!#AJK;GJK;GJKSML+SML+SA!!!!!!!!!!!!!0``!!!!!+#GJK;GJK;GL+SML+SML+!!!!!!!!!!!!!!``]!!!!!I+;GJK;GJK;ML+SML+SMI!!!!!!!!!!!!!$``Q!!!!#AJK;GJK;GJKSML+SML+SA!!!!!!!!!!!!!0``!!!!!+;GJK;GJK;GL+SML+SMJK9L+SM!!!!!!!!!``]!!!!!!+#AJK;GJK;ML+SMJK;A+SML+SML!!!!!!$``Q!!!!!!!!#AJK;GJKSMJK;A+SML+SML!!!!!!!!!0``!!!!!!!!!!!!I+;GJK;;+SML+SML+Q!!!!!!!!!!``]!!!!!!!!!!!!!!+#;+SML+SML+Q!!!!!!!!$`!!$``Q!!!!!!!!!!!!!!!!!!+SML+Q!!!!!!!!!!``]!!0``!!!!!!!!!!!!!!!!!!!!!!!!!!!!!!!!!!!!`Q!!``]!!!!!!!!!!!!!!!!!!!!!!!!!!!!!!!!!!!$`!!$``Q!!!!!!!!!!!!!!!!!!!!!!!!!!!!!!!!!!!0]!!0``!!!!!!!!!!!!!!!!!!!!!!!!!!!!!!!!!!!!`Q!!``]!!!!!!!!!!!!!!!!!!!!!!!!!!!!!!!!!!!$`!!$``Q!!!!!!!!!!!!!!!!!!!!!!!!!!!!!!!!!!````!0``!!!!!!!!!!!!!!!!!!!!!!!!!!!!!!!!!!!!!!!!````````````````````````````````````````````!!!!4!!!!!%!2!$RQOG`-1!!!!)(1WRB=X-A-1N$&lt;'&amp;T=S!R,G.U&lt;!!Q1&amp;!!!\"V$&lt;(6T&gt;'6S)'^G)'.M98.T)(\"S;8:B&gt;'5A:'&amp;U91!\"!!!!!!!Q!!!!!1!E1&amp;!!!\"V$&lt;(6T&gt;'6S)'^G)'.M98.T)(\"S;8:B&gt;'5A:'&amp;U91!$!!!!!!!!!!!!-!!\"2F\")5#&amp;&amp;&lt;8\"U?5.M98.T,GRW9WRB=X-[27VQ&gt;(F$&lt;'&amp;T=SZD&gt;'Q!!!!!!!!!!Q!!!&amp;!!!!!!!!!%\"!!!!!!!&amp;A!&amp;!#-!(A!!!\"9!!!!'!!!!)Q!!!\"Y!!!!!!1!!!!!!!!!!!!!!!!!!!!!!!!!!!!!!!!!!#A!!!!!!!!!%5'&amp;O:1!!!'E!!!!!!!!%\"!!!!!!!!Q!\"!\"!!C1!!!!-!!!!#!!!!%!!!!)E!!!!!!1!!!!!!!!!!!!!!!!!!!!!!!!!!!!!!!!!!#A!!!!!!!!!&gt;1WRV=X2F=C\"P:C\"D&lt;'&amp;T=S\"Q=GFW982F)'2B&gt;'%!!!!!!!\"1!!!!!!!!\"!1!!!!!!!%!!1!/!\"I!!!!\"!!!!!A!!!!Y!!!!;!!!!!!%!!!!!!!!!!!!!!!!!!!!!!!!!!!!!!!!!!!I!!!!!!!!!\"&amp;\"B&lt;G5!!!*X!!!&amp;&amp;HC=H:1`;\".2(-&gt;`\\Z,I3T$U*5WVQ5CCP,2&amp;UM7`.@CHVN?B5AI3#QY\"/RTI&amp;IJ5H&gt;LFFB1#!3'$U,&amp;:(4)I4E8C&gt;)O41TO%TCY/&amp;O8M8@S^/^`F'CY/8MDFXLXX_8X@\\`O_\"##7:J/;!ZMW%(;%$]MW*.AC0GT:-#%?J0=_*SH)KQ#&amp;9OYU`UC%G&gt;ZD3_1X!FHCE\"_:0,%\"?!(Y2?B?]B@4,&amp;WCCWR(=QD/H[5\\&lt;&amp;5SG3S/ZOEK/]#*H!VH^(W3@'3]\"Q,%_#,:\\F/P\"F[J&amp;5]GYE!;+1O!68\"L&amp;2MOO^6A5/?+W#&gt;%F?E@^Y_(SU\"]B2XC\\SGX8-+'[VD/K\"'=.W&lt;EH@=9@Z@D^6BXVC0(Y,ROHEM^:!XC;%^Y`C&gt;N&amp;'=VGH5,R'WY9;(7$(1[(&gt;[&lt;2F45Y:0(6P'T,MQ,GQI&amp;WBBQ.SX1&amp;$@F3MZ*L)LA/F2(9H-72)S;R\"2==O'%\"[/CK\\HFQ3,PP!H3NSS))NVKN23.['P6;F8KMB=+N?&gt;^^,E.:1NCP,?!;`P@U&amp;H]YNE?9L@@*4Y\"562?U]WJ6#;Y\\Y.C78-.DSL$&lt;Y=:(B&gt;V\"L+/*A]+NK8D#S==DQS;O#-&gt;LU'\\X=9G]#[&lt;E\"6/\\%39W;OB\"N[6PP]VU.0XU21/.U\"(&gt;.SX4Q^[=!`.&amp;\\]?0`.]5-'30KDB\"GQ&lt;JL&lt;'IL23H)ZQU3_7)])EO'9Y?'0`&amp;&lt;TII\"%W+HCE35JE6ZD*F[%'J%+$2UI)XC@.E6D[(]&amp;$P3&lt;#5P.6?0$'P?!&amp;[%$Q*-\\.%&lt;H,_,E,_KW/$.R&gt;\\W,O[,7BX%%!U@%)A\"ZVP`JPOMP_I`?(Q^`GD1`OU(&amp;&amp;*P]!ITNFNQ!!!!!)!!!!)!!!\"5A!!!!Q!!&amp;#2%B1)56N=(2Z1WRB=X-O&lt;(:D&lt;'&amp;T=TJ&amp;&lt;8\"U?5.M98.T,G.U&lt;!!!!!!!!!!$!!!!@!!!!*6YH'.A9*AI)-(UD[(O,Q/4Q&amp;=A1`IP!\\/A(_.P\"A:/0Y($1*J21*,Z(Y0M8Q&lt;W8QQ-ANJA'?UDOBQ-5+$+RKBCR?2SGIG\"1Z,DM#!(7!&amp;(CQ&lt;$````69I9Q2*@DVS$KT`C!W?W8!#2+L0E7X;!O@^!*)=%!&amp;UH)5E!!!!)!!!!\"Q!!!1!!!!$`!!!!\"!!!!\"J-6E.M98.T5(*J&gt;G&amp;U:52B&gt;'&amp;597*0=G2F=AABA!)!!!!#!!1!\"Q!-!%!!!@````]!!!!\"!!%!!!!!!!!!!!!!!\"N-6E.M98.T5(*J&gt;G&amp;U:52B&gt;'&amp;5;7VF=X2B&lt;8!))9!#!!!!!1!%!!=!!1!!QOG`-1!!!!!!!!!;4&amp;:$&lt;'&amp;T=V\"S;8:B&gt;'6%982B6(FQ:52F=W-))9!#!!!!!1!)!$$`````!!%!!!!!!!Y!!!!\"!!9!5!!!!!%!!!!!!!!!!!!?4&amp;:$&lt;'&amp;T=V\"S;8:B&gt;'6%982B2':M&gt;%2B&gt;'&amp;4;8JF##'!!A!!!!%!\"!!$!!%!!!!!!!!!!!!!!!!!!!1!!!\"!!!!!+!!!!!)!!!1!!!!!!1!!!!!!!!!!!!!!!!!!!!!!!!!!!!!!!!!!!!!!!!$`!!%!!A!$!!Y!!!$I!!Y%!!!!!!Y!ZQ$7!!!!\\Q!/\"!!!!!!/!/=!VA!!!09!$A1!!!!!$A$H!.9!!!!!!!!!!!!!!!!!!!!!!!!!!!!!!!!!!!!!!!!!!!!!!!!!!!!!!!!!!!!!!!!!!!!!!!!!!!!!!!!!!!!!!!!!!!!!!!!!!!!!!!!!!!!!!!!!!!!!!!!!!!!!!!!!!!!!!!!!!!!!!!!!!!!!!!!!!!!!!!!!!!!!!!!!!!!!!!!!!!!!!!!!!!!!!!!!!!!!!!!!!!!!!!!!!!!!!!!!`1!.B!#!!!!.!.!!O1:597BP&lt;7%'6'&amp;I&lt;WVB\"F2B;'^N91%R!&amp;*45E-.#A!$4&amp;:$1UR#6F=!!!`Y!!!$9!!!!#!!!!`9!!!!!!!!!!!!!!!A!!!!.!!!!!!!!!!84%F#4A!!!!!!!!%E4&amp;:45A!!!!!!!!%Y4%FW;1!!!!!!!!&amp;-1U^/5!!!!!!!!!&amp;A6%UY-!!!!!!!!!&amp;U2%:%5Q!!!!!!!!')4%FE=Q!!!!!!!!'=6EF$2!!!!!!!!!'Q&gt;G6S=Q!!!!!!!!(%35.04A!!!!!!!!(9;7.M/!!!!!!!!!(M1V\"$-A!!!!!!!!)!2&amp;2)5!!!!!!!!!)54%FG=!!!!!!!!!)I6&amp;*F9Q!!!!)!!!)]2F\")9A!!!!!!!!*Y2F\"421!!!!!!!!+-4%FC:!!!!!!!!!+A1E2)9A!!!!!!!!+U1E2421!!!!!!!!,)6EF55Q!!!!!!!!,=466*2!!!!!!!!!,Q3%F46!!!!!!!!!-%2F2\"1A!!!!!!!!-9!!!!!0````]!!!!!!!!!!$D'MAI!!!!!`````Q!!!!!!!!!=,-;S#A!!!!$`````!!!!!!!!!*!ARL)+!!!!!0````]!!!!!!!!\"\"\"4'MAI!!!!!`````Q!!!!!!!!&amp;E#-;S#A!!!!$`````!!!!!!!!!N$]R&lt;)+!!!!!0````]!!!!!!!!$&amp;0$&amp;MAI!!!!!`````Q!!!!!!!!.)Z-7S#A!!!!4`````!!!!!!!!!_T9R&lt;)+!!!!!0````]!!!!!!!!$`-T&amp;MAI!!!!!`````Q!!!!!!!!3!Q-7S#A!!!!$`````!!!!!!!!#)3UR&lt;)+!!!!!0````]!!!!!!!!)V+D&amp;MAI!!!!!`````Q!!!!!!!!E)H-7S#A!!!!,`````!!!!!!!!#4S1R&lt;)+!!!!!`````]!!!!!!!!*E)4&amp;MAI!!!!%`````Q!!!!!!!!I!?-7S#A!!!!$`````!!!!!!!!#F2MR&lt;)+!!!!!0````]!!!!!!!!-U'$&amp;MAI!!!!!`````Q!!!!!!!!T=6-7S#A!!!!$`````!!!!!!!!$2\")R&lt;)+!!!!!0````]!!!!!!!!.E$T&amp;MAI!!!!!`````Q!!!!!!!!W=--7S#A!!!!$`````!!!!!!!!$K!ER&lt;)+!!!!!0````]!!!!!!!!/K\"D&amp;MAI!!!#!`````Q!!!!!!!!\\5$-7S#A!!!!!</Property>\r\n   <Property Name=\"NI.LVClass.Geneology\" Type=\"Xml\"><String>\r\r\n<Name></Name>\r\r\n<Val>!!!!!1!!!!%327VQ&gt;(F$&lt;'&amp;T=SZM&gt;G.M98.T!&amp;\"53$!!!!!!!!!!!!!!!!%!!1!!!!!!!!!!!!%!\"A\"1!!!!!1!!!!!!!!!!!!!!!1Z-97*73568)%^C;G6D&gt;!\"16%AQ!!!!!!!!!!!!##'!!A!!!!!</Val>\r\r\n</String>\r\r\n</Property>\r\n   <Item Name=\"EmptyClass.ctl\" Type=\"Class Private Data\" URL=\"EmptyClass.lvclass/EmptyClass.ctl\">\r\n      <Property Name=\"NI.LibItem.Scope\" Type=\"Int\">2</Property>\r\n   </Item>\r\n</LVClass>\r\n"  # EmptyClass.lvclass
  n1 = property class="App"() -> ("App.Version"=w7:string)  [unwired: 2 in, 2 out]
  n2 = Match Pattern(string=w7, regular expression="^8.2") -> (offset past match=w16:i32)  [unwired: 1 in, 3 out]
  n3 = Match Pattern(string=w7, regular expression="^8.5") -> (offset past match=w13:i32)  [unwired: 1 in, 3 out]
  n4 = Match Pattern(string=w7, regular expression="^9") -> (offset past match=w6:i32)  [unwired: 1 in, 3 out]
  n5 = Greater Or Equal To 0?(x=w16) -> (x >= 0?=w12:bool)
  n6 = Greater Or Equal To 0?(x=w13) -> (x >= 0?=w11:bool)
  n7 = Greater Or Equal To 0?(x=w6) -> (x >= 0?=w5:bool)
  n8 = Or(x=w12, y=w11) -> (x .or. y?=w10:bool)
  n9 = Select(t="﻿<?xml version='1.0' encoding='UTF-8'?>\r\n<LVClass LVVersion=\"9006002\">\r\n\t<Property Name=\"NI.Lib.Icon\" Type=\"Bin\">#1\"A!A!!!!)!\"1!&amp;!!!-!%!!!@````]!!!!\"!!%!!!(]!!!*Q(C=\\&gt;8\"=&gt;MQ%!8143;(8.6\"2CVM#WJ\",7Q,SN&amp;(N&lt;!NK!7VM#WI\"&lt;8A0$%94UZ2$P%E\"Y.?G@I%A7=11U&gt;M\\7P%FXB^VL\\`NHV=@X&lt;^39O0^N(_&lt;8NZOEH@@=^_CM?,3)VK63LD-&gt;8LS%=_]J'0@/1N&lt;XH,7^\\SFJ?]Z#5P?=F,HP+5JTTF+5`Z&gt;MB$(P+1)YX*RU2DU$(![)Q3YW.YBG&gt;YBM@8'*\\B':\\B'2Z&gt;9HC':XC':XD=&amp;M-T0--T0-.DK%USWS(H'2\\$2`-U4`-U4`/9-JKH!&gt;JE&lt;?!W#%;UC_WE?:KH?:R']T20]T20]\\A=T&gt;-]T&gt;-]T?/7&lt;66[UTQ//9^BIHC+JXC+JXA-(=640-640-6DOCC?YCG)-G%:(#(+4;6$_6)]R?.8&amp;%`R&amp;%`R&amp;)^,WR/K&lt;75?GM=BZUG?Z%G?Z%E?1U4S*%`S*%`S'$;3*XG3*XG3RV320-G40!G3*D6^J-(3D;F4#J,(T\\:&lt;=HN+P5FS/S,7ZIWV+7.NNFC&lt;+.&lt;GC0819TX-7!]JVO,(7N29CR6L%7,^=&lt;(1M4#R*IFV][.DX(X?V&amp;6&gt;V&amp;G&gt;V&amp;%&gt;V&amp;\\N(L@_Z9\\X_TVONVN=L^?Y8#ZR0J`D&gt;$L&amp;]8C-Q_%1_`U_&gt;LP&gt;WWPAG_0NB@$TP@4C`%`KH@[8`A@PRPA=PYZLD8Y!#/7SO!!!!!!</Property>\r\n\t<Property Name=\"NI.Lib.Version\" Type=\"Str\">1.0.0.0</Property>\r\n\t<Property Name=\"NI.LVClass.ClassNameVisibleInProbe\" Type=\"Bool\">true</Property>\r\n\t<Property Name=\"NI.LVClass.FlattenedPrivateDataCTL\" Type=\"Bin\">#1\"A!A!!!!)!\"1!&amp;!!!-!%!!!@````]!!!!\"!!%!!\")D5F.31QU+!!.-6E.$4%*76Q!!$JQ!!!/(!!!!)!!!$HQ!!!!8!!!!!2*&amp;&lt;8\"U?5.M98.T,GRW9WRB=X-!!!!!?!E!9!)!-!!!+!!!!!!!!!1!!Q!]!,Q!(U!!!A!!!!!\"!!%!\"P````]!!!!!!!!!!!!!!!#!$C08/\"J'4&lt;*P]\".32^:Y!!!!$!!!!\"!!!!!!?WY#\"WJF0EK_^3U'=&amp;$!7N1&gt;D.G0!,)%[9!*G/TY1HY!!%!!!!!!!!!!!\"!!!!!!!!!!!!!!!!!!!!!!!!!!3Q!\"4&amp;:$1S&amp;&amp;&lt;8\"U?5.M98.T,GRW9WRB=X-[27VQ&gt;(F$&lt;'&amp;T=SZD&gt;'Q!!!!!!!%!!F:*4%)!!!!!5&amp;2)-!!!!!5!!1!\"!!!!!!)!!Q!!!!!#!!%!!!!!!\"9!#1!#%!!1!2!!%!11!\"!!%!!Q!\"!!!!!!!!!^!!!\"%(C=9W$!\"0_\"!%AR-D!QNQ\"J&gt;CTC)#Y,&amp;KU5![A&gt;''R]9JC!%;C'[1M$V+%1Q)T+\"1)W,$I\"IDY7C1!!!!!!!$!!!6:*2&amp;-B27VQ&gt;(F$&lt;'&amp;T=SZM&gt;G.M98.T/E6N=(2Z1WRB=X-O9X2M!!!!!!!!!!-!!!\"Y!!!!N(C==W2A9-AUND#L9%#!Z0S56\"#^!)B@-]4(256'RR[?%.K&gt;I])2(\"A5&amp;L[$%3C\"+&gt;R&gt;SL\"$#SD4[;;R1QF-/_RQ\".-OI3^!ZP7GK,$!N'5!_1?\"ZI#-_A]%)(F'\"G9'@Y:QBHAENTD\\O\\AC==&amp;O!A!U13&gt;:!!!!$1E!9!)!!!5Z,D\"C-A!!!!!!!!#!`````Y!!!!'!!!!\"A!!!!9!!!!'!!!!\"A!!!!9!!!!'!!!!\"A!!!!9!!!!'!!!!\"A'!!!9'9!!''\"A!\"G!'!!;!!1!'Q!-!\"L!.!!;-/Q!'A^5!\"I#L!!;!V1!'A+M!\"I$6!!;!KQ!'A.5!\"G#O!!99W!!'\"O!!\"A'!!!@````]!!!1!````````````````````````````````````````````!!!!!!!!!!!!!!!!!!!!!!!!!!!!!!!!!!!!!!!!``]!!!!!!!!!!!!!!!!!!!!!!!!!!!!!!!!!!!!!!!$``Q!!!!!!!!!!!!!!!!!!!!!!!!!!!!!!!!!!!!!!!0``!!!!!!!!!!!!!!!!!!!!!!!!!!!!!!!!!!!!!!!!``]!!!!!!!!!!!!!!!!!!!!!!!!!!!!!!!!!!!!!!!$``Q!!!!!!!!!!!!!!!!!!!!!!!!!!!!!!!!!!!!!!!0``!!!!!!!!!!!!!!!!!!!!!!!!!!!!!!!!!!!!!!!!``]!!!!!!!!!!!!!!!!!!!!!!!!!!!!!!!!!!!!!!!$``Q!!!!!!!!!!!!!!!!!!!!!!!!!!!!!!!!!!!!!!!0``!!!!!!!!!!!!!!!!!!!!!!!!!!!!!!!!!!!!!!!!``]!!!!!!!!!!!!!!!!!!!!!!!!!!!!!!!!!!!!!!!$``Q!!!!!!!!!!?(A!!!!!!!!!!!!!!!!!!!!!!!!!!0``!!!!!!!!?+SKK[RY!!!!!!!!!!!!!!!!!!!!!!!!``]!!!!!?+SKI[/DI[OM?!!!!!!!!!!!!!!!!!!!!!$``Q!!?+SKI[/DI[/DI[/LL(A!!!!!!!!!!!!!!!!!!0``!+OKI[/DI[/DI[/DI[/DK[Q!!!!!!!!!!!!!!!!!``]!KKKDI[/DI[/DI[/DI[0_KQ!!!!!!!!!!!!!!!!$``Q#KK[OKI[/DI[/DI[0_`P[K!!!!!!!!!!!!!!!!!0``!+KLK[OLKK/DI[0_`P\\_`KI!!!!!!!!!!!!!!!!!``]!KKOLK[OLK[KM`P\\_`P\\_KA!!!!!!!!!!!!!!!!$``Q#KK[OLK[OLK`\\_`P\\_`P[K!!!!!!!!!!!!!!!!!0``!+KLK[OLK[OL`P\\_`P\\_`KI!!!!!!!!!!!!!!!!!``]!KKOLK[OLK[P_`P\\_`P\\_KA!!!!!!!!!!!!!!!!$``Q#KK[OLK[OLK`\\_`P\\_`P[K!!!!!!!!!!!!!!!!!0``!+KLK[OLK[OL`P\\_`P\\_`KI!!!!!!!!!!!!!!!!!``]!K[OLK[OLK[P_`P\\_`P[LKQ!!!!!!!!!!!!!!!!$``Q!!J+KLK[OLK`\\_`P[LL+1!!!!!!!!!!!!!!!!!!0``!!!!!+3LK[OL`P[LK[1!!!!!!!!!!!!!!!!!!!!!``]!!!!!!!#EK[OLK[-!!!!!!!!!!!!!!!!!!!!!!!$``Q!!!!!!!!!!J+-!!!!!!!!!!!!!!!!!!!!!!!!!!0```````````````````````````````````````````Q!!!!)!!1!!!!!!-!!\"2F\")5#&amp;&amp;&lt;8\"U?5.M98.T,GRW9WRB=X-[27VQ&gt;(F$&lt;'&amp;T=SZD&gt;'Q!!!!!!!!!!Q!!!FM!!!4*?*SN6-VL%U%=`5V=:2)MG8SI87R*,*/W3(,RMQ;DJ:U?+K5IM?#B9)-&lt;0[!VUM4KK&lt;XM*96#1=B\"[-&amp;,LBZS]#I34XPRZ-%?FPY(8IK#X9W`W72XUV8CR6V9BNVZ\\`XGP==#+*`:=-C'41M)/]4&amp;AA52T3!!\\2S&amp;XM77S#]A3:69-%W8W(\\)*C-7H.;-=8J&amp;V/&amp;\\&lt;SMJE(@M!,??9CIS23S);M;ZW\"VO-PZ_B.&gt;0OJ22/-^WC\"V[Q&amp;-`[)Z?1481*_5TFC-W%(&amp;\"5@3RO[8H::X,N_%=62X+M!6-'%-&lt;X*R!2J4_Z&amp;#38:*&amp;[2YF)/5EN&amp;IN(R4LAM;&gt;-;911\\,/O,M$-((%P/*GVM&amp;%(!TK&amp;&amp;Q&gt;E&lt;,@S.EF+!B.=+0+493^&gt;JX*OF)C:5X`&amp;@&lt;5AC1X:[B+$\\2P:/C?`A%)E0:$,Y49IAT\"W2P(($*ZQIKY,FJQ54&gt;#+URRX;X#NJ/#YK:Q5[9QY[11&amp;H5'@AT&lt;`YSB049[O`KS7COPJSO0UY^73^6K_M8[MYV3L:T73L83HQ%6B+&amp;?FK?89NVO*%#\"#KTUGVW\":L/*\"O$4B^Z#;)+&lt;(C\\KH%&lt;T$.&gt;]Z[3K\\^RN&gt;%\\]P0^%OJ@*BZS_AN`53^D57$)YT&lt;'G8PX`4&lt;UGD.(.1&amp;.B'?_V!;W\\XA8Z4=8^!'OQ0!!TB:CN`K:W66S&gt;15W^)1RWP+I3'[BKI^%)6D8P665BJ&amp;N6`5PHK(-5,#S%&amp;`MGJ`OUG*EYQ57(KI%0&lt;![:NSQY)W&lt;D(^G]\\$K&gt;JX.M$S0%`]Z:OE=0WV]^]P;#N_2P5X4Y.STH59A!!!!!\"!!!!#!!!!!%!!!!1!!!!$!!!5*%3&amp;!B27VQ&gt;(F$&lt;'&amp;T=SZM&gt;G.M98.T/E6N=(2Z1WRB=X-O9X2M!!!!!!!!!!-!!!\"G!!!!&gt;HC=9W\"A+\"+190L(50?8A5HA+Z!B`:?\"7&gt;#0]4=$![?@Q'%AT3AA#237`=P!,KA.&amp;N9_IMP\"!!7K&lt;)QO6IS-(*)=BQ5ZQ,)=,2I-````Z`B[Z\"J=V2%@/&amp;.FFDS(\"!\"JMRG%!!!!!!!%!!!!\"Q!!!:1!!!!'!!!!)6^O;6^-98.U3WZP&gt;WZ0&gt;WZJ&lt;G&gt;-6E.M98.T1WRV=X2F=AE!9!)!!!!\"!!A!-0````]!!1!!!!!!$A!!!!%!\"A\"1!!!!!1!!!!!!!!!!!\"J-6E.M98.T5(*J&gt;G&amp;U:52B&gt;'&amp;597*0=G2F=AE!9!)!!!!#!!5!\"Q!!$!\"!!!(`````!!!!!1!\"!!!!!!!!!!!!!!!&lt;4&amp;:$&lt;'&amp;T=V\"S;8:B&gt;'6%982B6'FN:8.U97VQ#1\"A!A!!!!%!\"1!(!!!\"!!$&amp;O$7G!!!!!!!!!#:-6E.M98.T5(*J&gt;G&amp;U:52B&gt;'&amp;-98.U18\"Q&lt;'FF:&amp;2J&lt;76T&gt;'&amp;N=!E!9!)!!!!\"!!5!\"Q!!!1!!R&lt;AVJA!!!!!!!!!;4&amp;:$&lt;'&amp;T=V\"S;8:B&gt;'6%982B6(FQ:52F=W-*!'!#!!!!!1!)!$$`````!!%!!!!!!!Y!!!!\"!!9!5!!!!!%!!!!!!!!!!!!?4&amp;:$&lt;'&amp;T=V\"S;8:B&gt;'6%982B2':M&gt;%2B&gt;'&amp;4;8JF#1\"A!A!!!!%!\"1!$!!!\"!!!!!!!!!!!!!!!!!!1!!A!,!!!!\"!!!!%!!!!!I!!!!!A!!\"!!!!!!\"!!!!!!!!!!!!!!!!!!!!!!!!!!!!!!!!!!!!!!!!!DI!!!/\"?*S.5]NSUU!1&lt;%?7YW@C/![\"P$!1),T#_[\\#RF5_E,BM!V?5X66+67ONU+Z3.C?K_\"?_A2`AA\\BT9&amp;;SSTFSUGR0TWT0&lt;!P!'YTQZ`?PNT]\"L,8?4W-T\\UJ@[V.ZR?RXYRL%D-3*.Q1/OT,62C1&gt;&amp;81S6C&gt;/QCP@C!\\XD9]K'&amp;$YCQ*=/+!DJ_9PM99SPF\"5*W2)*Q@&amp;H)I4IF;]&gt;4C\"P%4:__[IE=E\"I1)U[5I([V2&gt;=6)?Y0B`*&amp;C/QQ/_C-RM'3GZD-4-I%6+3K3C2KI;W-$G1N&amp;45J2(%YJ+_%'-49]GY%Q.)CZG1-ULQ1XDLIKQZ&lt;GI[8H%?K'/J4]HKIM+^5`]DVJQILII\"N)X1-/D&gt;ER&amp;:_H5(GAOQC^\\Y`069@*B1\"7U(;\\(XY\"N+KZTLDYHI2&amp;&gt;R17Q4V#&lt;I$-BC*.?@\"K-D:_9.%9O*&gt;3E-73_55EGJ2TK-@/FH^BO$OIK\\N'3TI.!#W.,(.4-.738A#UR%]RC1Z-MY%SAE+:H:47I\\4J4]8QEPG&lt;TO6,2&amp;@2K^/;\"5$E7^=+JTD6:\\D\"2&lt;-\"HW#&amp;AQQ,^2%V(*L*9RKJ/1]VEHZ;A14*=..-IJ1XW1SF&amp;]GZO2#[XKN/,S4Q7&gt;G`9][SLCEV'BF$4,L6&gt;4H;1:VKLT%1N=U&gt;ZLLX+74(,L%?_/%1&lt;/\\C\"8&gt;T%,?RB(Q?%(?%W/LC$O\\C(9^T(!TQE`T\\#9TQBVTT$+:\\DR=,T\"8*^-8-]MJ_BB#;WS(0&lt;?)88Z+D;0[*MR)-!!!!!!&amp;]!!1!#!!-!\"!!!!%A!$11!!!!!$1$1!,E!!!\"0!!U%!!!!!!U!U!#Z!!!!6A!.\"!!!!!!.!.!!O1!!!&amp;W!!)1!A!!!$1$1!,E'6'&amp;I&lt;WVB\"F2B;'^N91:597BP&lt;7%\"-!\"35V*$$1I!!UR71U.-1F:8!!!/H!!!!Y=!!!!A!!!/@!!!!!!!!!!!!!!!)!!!!$1!!!.Y!!!!'5R*1EY!!!!!!!!\"0%R75V)!!!!!!!!\"5&amp;*55U=!!!!!!!!\":%R*&gt;GE!!!!!!!!\"?%.04F!!!!!!!!!\"D&amp;2./$!!!!!!!!!\"I%2'2&amp;-!!!!!!!!\"N%R*:(-!!!!!!!!\"S&amp;:*1U1!!!!!!!!\"X(:F=H-!!!!!!!!\"]%F$4UY!!!!!!!!#\"'FD&lt;$A!!!!!!!!#'%.11T)!!!!!!!!#,%R*:H!!!!!!!!!#1%:13')!!!!!!!!#6%:15U5!!!!!!!!#;%F15V)!!!!!!!!#@%R*9G1!!!!!!!!#E%*%3')!!!!!!!!#J%*%5U5!!!!!!!!#O&amp;:*6&amp;-!!!!!!!!#T%253&amp;!!!!!!!!!#Y%V6351!!!!!!!!#^%B*5V1!!!!!!!!$#&amp;:$6&amp;!!!!!!!!!$(%:515)!!!!!!!!$-!!!!!$`````!!!!!!!!!!!!!!!!!!!!!!!!!!!!!!!!!!!!(!!!!!!!!!!!`````Q!!!!!!!!#9!!!!!!!!!!$`````!!!!!!!!!+Q!!!!!!!!!!0````]!!!!!!!!!`!!!!!!!!!!!`````Q!!!!!!!!%%!!!!!!!!!!$`````!!!!!!!!!3!!!!!!!!!!!0````]!!!!!!!!\":!!!!!!!!!!!`````Q!!!!!!!!'9!!!!!!!!!!4`````!!!!!!!!!B1!!!!!!!!!!0````]!!!!!!!!#+!!!!!!!!!!!`````Q!!!!!!!!+M!!!!!!!!!!$`````!!!!!!!!\"L!!!!!!!!!!!0````]!!!!!!!!'O!!!!!!!!!!!`````Q!!!!!!!!&lt;M!!!!!!!!!!$`````!!!!!!!!#5Q!!!!!!!!!!0````]!!!!!!!!*6!!!!!!!!!!!`````Q!!!!!!!!F=!!!!!!!!!!$`````!!!!!!!!#:!!!!!!!!!!!0````]!!!!!!!!*`!!!!!!!!!!!`````Q!!!!!!!!I%!!!!!!!!!!$`````!!!!!!!!#ZQ!!!!!!!!!!0````]!!!!!!!!,J!!!!!!!!!!!`````Q!!!!!!!!OM!!!!!!!!!!$`````!!!!!!!!#^A!!!!!!!!!A0````]!!!!!!!!/'!!!!!!/27VQ&gt;(F$&lt;'&amp;T=SZD&gt;'Q!!!!!</Property>\r\n\t<Property Name=\"NI.LVClass.Geneology\" Type=\"Xml\"><String>\r\r\n<Name></Name>\r\r\n<Val>!!!!!2*&amp;&lt;8\"U?5.M98.T,GRW9WRB=X-!5&amp;2)-!!!!!!!!!!!!!!!!1!\"!!!!!!!!!!!!!!%!\"A\"1!!!!!1!!!!!!!!!!!!!\"$ERB9F:*26=A4W*K:7.U!&amp;\"53$!!!!!!!!!!!!!*!'!#!!!!!!!!!!!!!!</Val>\r\r\n</String>\r\r\n</Property>\r\n\t<Property Name=\"NI.LVClass.IsTransferClass\" Type=\"Bool\">false</Property>\r\n\t<Item Name=\"EmptyClass.ctl\" Type=\"Class Private Data\" URL=\"EmptyClass.ctl\">\r\n\t\t<Property Name=\"NI.LibItem.Scope\" Type=\"Int\">2</Property>\r\n\t</Item>\r\n</LVClass>\r\n", s=w5, f="﻿<?xml version='1.0' encoding='UTF-8'?>\n<LVClass LVVersion=\"8608001\">\n\t<Property Name=\"NI.Lib.Icon\" Type=\"Bin\">#'#!!1!!!!)!\"1!&amp;!!!-!%!!!@````]!!!!\"!!%!!!(]!!!*Q(C=\\&gt;8\"=&gt;MQ%!8143;(8.6\"2CVM#WJ\",7Q,SN&amp;(N&lt;!NK!7VM#WI\"&lt;8A0$%94UZ2$P%E\"Y.?G@I%A7=11U&gt;M\\7P%FXB^VL\\`NHV=@X&lt;^39O0^N(_&lt;8NZOEH@@=^_CM?,3)VK63LD-&gt;8LS%=_]J'0@/1N&lt;XH,7^\\SFJ?]Z#5P?=F,HP+5JTTF+5`Z&gt;MB$(P+1)YX*RU2DU$(![)Q3YW.YBG&gt;YBM@8'*\\B':\\B'2Z&gt;9HC':XC':XD=&amp;M-T0--T0-.DK%USWS(H'2\\$2`-U4`-U4`/9-JKH!&gt;JE&lt;?!W#%;UC_WE?:KH?:R']T20]T20]\\A=T&gt;-]T&gt;-]T?/7&lt;66[UTQ//9^BIHC+JXC+JXA-(=640-640-6DOCC?YCG)-G%:(#(+4;6$_6)]R?.8&amp;%`R&amp;%`R&amp;)^,WR/K&lt;75?GM=BZUG?Z%G?Z%E?1U4S*%`S*%`S'$;3*XG3*XG3RV320-G40!G3*D6^J-(3D;F4#J,(T\\:&lt;=HN+P5FS/S,7ZIWV+7.NNFC&lt;+.&lt;GC0819TX-7!]JVO,(7N29CR6L%7,^=&lt;(1M4#R*IFV][.DX(X?V&amp;6&gt;V&amp;G&gt;V&amp;%&gt;V&amp;\\N(L@_Z9\\X_TVONVN=L^?Y8#ZR0J`D&gt;$L&amp;]8C-Q_%1_`U_&gt;LP&gt;WWPAG_0NB@$TP@4C`%`KH@[8`A@PRPA=PYZLD8Y!#/7SO!!!!!!</Property>\n\t<Property Name=\"NI.Lib.Version\" Type=\"Str\">1.0.0.0</Property>\n\t<Property Name=\"NI.LVClass.ClassNameVisibleInProbe\" Type=\"Bool\">true</Property>\n\t<Property Name=\"NI.LVClass.FlattenedPrivateDataCTL\" Type=\"Bin\">#'#!!1!!!!)!\"1!&amp;!!!-!%!!!@````]!!!!\"!!%!!\"#&lt;5F.31QU+!!.-6E.$4%*76Q!!$41!!!.H!!!!)!!!$21!!!!8!!!!!2*&amp;&lt;8\"U?5.M98.T,GRW9WRB=X-!!!!!?!BAA!%!-!!!#!!!!!!!!!1!!Q!]!,Q!(U!!!A!!!!!\"!!%!\"P````]!!!!!!!!!!!!!!!$IV#HT8S013ZP9F?D765@+!!!!$!!!!\"!!!!!!&gt;B_ITDR1=U;^[EI:D:NBJ&gt;1&gt;D.G0!,)%[9!*G/TY1HY!!%!!!!!!!!!!!\"!!!!!!!!!!!!!!!!!!!!!!!!!!3Q!\"4&amp;:$1S&amp;&amp;&lt;8\"U?5.M98.T,GRW9WRB=X-[27VQ&gt;(F$&lt;'&amp;T=SZD&gt;'Q!!!!!!!%!!F:*4%)!!!!!5&amp;2)-!!!!!5!!1!\"!!!!!!)!!Q!!!!!#!!%!!!!!!\"Q!$!!#%!!1!2!!%!11!\"!!-!!1!\"!!%!!Q!\"!!!!!!11!!!22YH'.AQ!E9'2B9/)!U&amp;UTA0R\"!R*F\"8\"&lt;=7ME(5$MQW0D%M!!\"#-5)6-PUB1(K9!BA2O5#!2O;:A#'Z2)F!!!!!!!!-!!\"6EF%5S&amp;&amp;&lt;8\"U?5.M98.T,GRW9WRB=X-[27VQ&gt;(F$&lt;'&amp;T=SZD&gt;'Q!!!!!!!!!!Q!!!*]!!!$I?*T,9W\"AS$3W-&amp;P&amp;A!$*_3GJ)0I+%(?_W'=)IAJYDDPI#!*:!;(&gt;LAT`\"8J46$BM19J+W8?!K--4`D_9-'&amp;#@&amp;R5:(4MY1GBX4EK(-'\"17(B/RC\"MJD#X;5-/]*\"\"LNJ\\&amp;!!UQY\\]M#U3Q:)2_A,E+EA7W\"[:Y&amp;M!5K\":0]$!5C?E9'&amp;1:GBBK'&amp;I1@*`=\\_,KZ)8,!`!\"#T.X9!!!!!#QBAA!%!!!-Y,D9!!!!!!)$`````A!!!!9!!!!'!!!!\"A!!!!9!!!!'!!!!\"A!!!!9!!!!'!!!!\"A!!!!9!!!!'!9!!\"A:A!!99'!!'9!9!\"I!\"!!&lt;!!Q!'M!U!\"IQ\\!!;$V1!'A+M!\"I$6!!;!KQ!'A.5!\"I#L!!;!V1!'9+Y!\"BD9!!9'Y!!'!9!!\"`````Q!!\"!$```````````````````````````````````````````]!!!!!!!!!!!!!!!!!!!!!!!!!!!!!!!!!!!!!!!$``Q!!!!!!!!!!!!!!!!!!!!!!!!!!!!!!!!!!!!!!!0``!!!!!!!!!!!!!!!!!!!!!!!!!!!!!!!!!!!!!!!!``]!!!!!!!!!!!!!!!!!!!!!!!!!!!!!!!!!!!!!!!$``Q!!!!!!!!!!!!!!!!!!!!!!!!!!!!!!!!!!!!!!!0``!!!!!!!!!!!!!!!!!!!!!!!!!!!!!!!!!!!!!!!!``]!!!!!!!!!!!!!!!!!!!!!!!!!!!!!!!!!!!!!!!$``Q!!!!!!!!!!!!!!!!!!!!!!!!!!!!!!!!!!!!!!!0``!!!!!!!!!!!!!!!!!!!!!!!!!!!!!!!!!!!!!!!!``]!!!!!!!!!!!!!!!!!!!!!!!!!!!!!!!!!!!!!!!$``Q!!!!!!!!!!!!!!!!!!!!!!!!!!!!!!!!!!!!!!!0``!!!!!!!!!!\"Y?!!!!!!!!!!!!!!!!!!!!!!!!!!!``]!!!!!!!\"YL+KLL(A!!!!!!!!!!!!!!!!!!!!!!!$``Q!!!!\"YL+KDI[/DK[RY!!!!!!!!!!!!!!!!!!!!!0``!!\"YL+KDI[/DI[/DI[OM?!!!!!!!!!!!!!!!!!!!``]!K[KDI[/DI[/DI[/DI[/LL!!!!!!!!!!!!!!!!!$``Q#KKK/DI[/DI[/DI[/DI`[L!!!!!!!!!!!!!!!!!0``!+KLK[KDI[/DI[/DI`\\_`KI!!!!!!!!!!!!!!!!!``]!KKOLK[OKI[/DI`\\_`P\\_KA!!!!!!!!!!!!!!!!$``Q#KK[OLK[OLKKT_`P\\_`P[K!!!!!!!!!!!!!!!!!0``!+KLK[OLK[OL`P\\_`P\\_`KI!!!!!!!!!!!!!!!!!``]!KKOLK[OLK[P_`P\\_`P\\_KA!!!!!!!!!!!!!!!!$``Q#KK[OLK[OLK`\\_`P\\_`P[K!!!!!!!!!!!!!!!!!0``!+KLK[OLK[OL`P\\_`P\\_`KI!!!!!!!!!!!!!!!!!``]!KKOLK[OLK[P_`P\\_`P\\_KA!!!!!!!!!!!!!!!!$``Q#LK[OLK[OLK`\\_`P\\_`KOL!!!!!!!!!!!!!!!!!0``!!#EKKOLK[OL`P\\_`KOMJ!!!!!!!!!!!!!!!!!!!``]!!!!!J+OLK[P_`KOLJ!!!!!!!!!!!!!!!!!!!!!$``Q!!!!!!!+3LK[OLIQ!!!!!!!!!!!!!!!!!!!!!!!0``!!!!!!!!!!#EIQ!!!!!!!!!!!!!!!!!!!!!!!!!!````````````````````````````````````````````!!!!!A!\"!!!!!!!%!!)!$A!!!$!!!5:13&amp;!B27VQ&gt;(F$&lt;'&amp;T=SZM&gt;G.M98.T/E6N=(2Z1WRB=X-O9X2M!!!!!!!!!!-!!!)Z!!!%P8C=N6*.;\".\"&amp;(Y4JTIJ\"':LQ#YE:AW4NG\"TUI-)IL4&lt;1[55*29]&amp;(2R5R7+E3:74_VF,TE5#E)I1A^?=P71AXA4]&lt;9?0(FI$UO0XE1M,ND&gt;^=VM9\\;BR8BQBPFZ\\XXTXMQX(Q\"^RU&gt;4);TZ@\"_8O=\"W#1!N]Q8S#UB7*Q&amp;&lt;Y,OJE/1Q-M9OGUXYBN%^D*\\G/JY92P]Z\\;&lt;QO(C4%]UB$'[1-(68&amp;([S$;?'S=#:E,.7*C%1]Q+F4P'7^;4K#/F.FZGO]K2^U]WM#G]=UW#2$\\U]A(EGI.0J^#((6-%L@Q%_&amp;^[E!AZXA79B@#GP*J&amp;^?/(7B9@9&amp;TVM=/.9\\#.@?&amp;.-:XPW$MH=&gt;NY#!5,P;@/3.159#5REMH16?!7N3O#YK@O=(F*(%^2.+?L3:J0$!.R^,/;HFZ`6'^56I\\:E0&amp;CW[H8D[=LD6;N2.7SL92X$KHZ*PEF75&amp;_8)+M'\\89&lt;HY6T%H^7?%@!3*D&gt;)U(G4Z*A_H=?3C,E5[6I)#E9,@N@\":.@'V1Q%DG190,L`S)9U_5H+;&lt;6;JWE'%J)L\"DH=X11(2TK\"N,TC9OR869JD:]3:M4UPA#@Q84LA4E^]HYI5]K&gt;Y&lt;/R[EB)@N!CFJBF-XQ&lt;PY$Y&lt;*PNUS^U4LQKM&amp;&amp;AU'X818)*Z\"JZ$3HFY8!?\\5US#2I/:&amp;`OS3:IW#63\\LPN9P26L1X9CK.Y?AOS1'%2/U@&lt;\"DP[`M?4K+\"M$1?I/&lt;&lt;C()P+KVKUIR9$?X)^WD\\^\"ERT26!!!!!!!!!)!!!!)!!!\"M=!!!!Q!!&amp;#2%B1)56N=(2Z1WRB=X-O&lt;(:D&lt;'&amp;T=TJ&amp;&lt;8\"U?5.M98.T,G.U&lt;!!!!!!!!!!$!!!!9A!!!(&gt;YH'.A9#A7E'$[RV$X6_!LE*,_)?D(_*O\"A&gt;.0Y$#1:B31\"!L+`B85\"ANKM_CKMD'K7$&amp;T3()=&amp;O1!CX'U;$$]``^@J9C2YSP,.29@F6HS(\")-D!T-$,C\"$!!%?R?U!!!!!!!)!!!!\"Q!!!8I!!!&amp;&amp;!!!!\"1!!!\"J-6E.M98.T5(*J&gt;G&amp;U:52B&gt;'&amp;597*0=G2F=ABAA!%!!!!#!!5!\"Q!!$!\"!!!(`````!!!!!1!\"!!!!!!!!!!!!!!!&lt;4&amp;:$&lt;'&amp;T=V\"S;8:B&gt;'6%982B6'FN:8.U97VQ#'#!!1!!!!%!\"1!(!!!\"!!$%PY+A!!!!!!!!!#:-6E.M98.T5(*J&gt;G&amp;U:52B&gt;'&amp;-98.U18\"Q&lt;'FF:&amp;2J&lt;76T&gt;'&amp;N=!BAA!%!!!!\"!!5!\"Q!!!1!!R,_#I!!!!!!!!!!;4&amp;:$&lt;'&amp;T=V\"S;8:B&gt;'6%982B6(FQ:52F=W-)9)!\"!!!!!1!)!$$`````!!%!!!!!!!Y!!!!\"!!9!5!!!!!%!!!!!!!!!!!!?4&amp;:$&lt;'&amp;T=V\"S;8:B&gt;'6%982B2':M&gt;%2B&gt;'&amp;4;8JF#'#!!1!!!!%!\"1!$!!!\"!!!!!!!!!!!!!!!!!!!!!!1!!!\"!!!!!+!!!!!)!!!1!!!!!!1!!!!!!!!!!!!!!!!!!!!!!!!!!!!!!!!!!!!!!!!%6!!!\"S8C=D9`*3A.\"&amp;%60&gt;W7U.=9Y4^!,FS+Y%R=3#),,E#_Q[5'%FAZ**=2&gt;U)W@Y:_Y]80=_!@?&gt;(==&gt;H+B[LZ8&lt;TA&amp;($0A]`XN[26Q/^=01`P93Y0R_#S&gt;BIO\\^3M6WJ4,&lt;F^.P81SNP()TR)`L`+(I`NJ9'-`#GT!#C%Y(V3I9F!9;@AZ,AVOZ6;6[3MS+MB,O=#BW;VDEP3/2H&gt;OMI%N%H'7U.:+1VX&gt;44/*%E\\_A\\#I-6%3F=\\/FCZ,FS[?74ICK9H#%^5;,&gt;:,IF-2V8B7PK\"XJ?,F2C_&amp;?`HG*`_KCQ[(]J=6LD4\\C&amp;VJLZ3&lt;[W`U%S_VH[P9[X#A39BLY;NC;L-B[EWWW';(1WXQ],Y!-/J$?!!!!!!!!&amp;]!!1!#!!-!\"!!!!%A!$A1!!!!!$A$H!.9!!!\"0!!Y%!!!!!!Y!ZQ$7!!!!6A!/\"!!!!!!/!/=!VA!!!&amp;W!!)1!A!!!$A$H!.9'6'&amp;I&lt;WVB\"F2B;'^N91:597BP&lt;7%\"-!\"35V*$$1I!!UR71U.-1F:8!!!..!!!!W=!!!!A!!!.&amp;!!!!!!!!!!!!!!!)!!!!$1!!!.9!!!!'%R*1EY!!!!!!!!\"-%R75V)!!!!!!!!\"2&amp;*55U=!!!!!!!!\"7%R*&gt;GE!!!!!!!!\"&lt;%.04F!!!!!!!!!\"A&amp;2./$!!!!!!!!!\"F%2'2&amp;-!!!!!!!!\"K%R*:(-!!!!!!!!\"P&amp;:*1U1!!!!!!!!\"U(:F=H-!!!!!!!!\"Z%F$4UY!!!!!!!!\"_'FD&lt;$A!!!!!!!!#$%.11T)!!!!!!!!#)%253&amp;!!!!!!!!!#.%R*:H!!!!!!!!!#3%:13'-!!!!!!!!#8%:15U5!!!!!!!!#=%R*9G1!!!!!!!!#B%*%3'-!!!!!!!!#G%*%5U5!!!!!!!!#L&amp;:*6&amp;-!!!!!!!!#Q%V6351!!!!!!!!#V%B*5V1!!!!!!!!#[&amp;:$6&amp;!!!!!!!!!#`%:515)!!!!!!!!$%!!!!!$`````!!!!!!!!!!!!!!!!!!!!!!!!!!!!!!!!!!!!(!!!!!!!!!!!`````Q!!!!!!!!#9!!!!!!!!!!$`````!!!!!!!!!+Q!!!!!!!!!!0````]!!!!!!!!!`!!!!!!!!!!!`````Q!!!!!!!!%%!!!!!!!!!!$`````!!!!!!!!!31!!!!!!!!!!0````]!!!!!!!!\"&lt;!!!!!!!!!!!`````Q!!!!!!!!'A!!!!!!!!!!4`````!!!!!!!!!E1!!!!!!!!!!0````]!!!!!!!!#6!!!!!!!!!!!`````Q!!!!!!!!,9!!!!!!!!!!$`````!!!!!!!!\"NQ!!!!!!!!!!0````]!!!!!!!!'Z!!!!!!!!!!!`````Q!!!!!!!!&lt;M!!!!!!!!!!$`````!!!!!!!!\"S!!!!!!!!!!!0````]!!!!!!!!*9!!!!!!!!!!!`````Q!!!!!!!!FM!!!!!!!!!!$`````!!!!!!!!#;!!!!!!!!!!!0````]!!!!!!!!+#!!!!!!!!!!!`````Q!!!!!!!!I5!!!!!!!!!!$`````!!!!!!!!#W!!!!!!!!!!!0````]!!!!!!!!,;!!!!!!!!!!!`````Q!!!!!!!!O5!!!!!!!!!)$`````!!!!!!!!$,!!!!!!$E6N=(2Z1WRB=X-O9X2M!!!!!!</Property>\n\t<Property Name=\"NI.LVClass.Geneology\" Type=\"Xml\"><String>\n\n<Name></Name>\n\n<Val>!!!!!2*&amp;&lt;8\"U?5.M98.T,GRW9WRB=X-!5&amp;2)-!!!!!!!!!!!!!!!!1!\"!!!!!!!!!!!!!!%!\"A\"1!!!!!1!!!!!!!!!!!!!\"$ERB9F:*26=A4W*K:7.U!&amp;\"53$!!!!!!!!!!!!!)9)!\"!!!!!!!!!!!!!!</Val>\n\n</String>\n\n</Property>\n\t<Item Name=\"EmptyClass.ctl\" Type=\"Class Private Data\" URL=\"EmptyClass.ctl\">\n\t\t<Property Name=\"NI.LibItem.Scope\" Type=\"Int\">2</Property>\n\t</Item>\n</LVClass>") -> (s? t:f=w2:string)
  n10 = Not A Number/Path/Refnum?(number/path/refnum="Project Item To Create Class Below(Use MyComputer if not wired)") -> (NaN/Path/Refnum?=w23:bool)
  n11 = Select(t=w9, s=w10, f=w2) -> ()  [unwired: 1 out]
  n12 = case shown="No Error" "error in (no error)" {
    selector: "error in (no error)" -> [w54 w123]
    tunnel: [w36 w123] -> w25
    tunnel: "Project Refnum In" -> [w48 w122]
    tunnel: w23 -> [w51 _]
    tunnel: "Project Item To Create Class Below(Use MyComputer if not wired)" -> [w53 _]
    tunnel: [w48 w122] -> w21
    tunnel: "ClassName" -> [w30 _]
    tunnel: "ClassFolder" -> [w35 _]
    tunnel: [w38 _] -> w17
    tunnel: [w44 _] -> w18
    tunnel: [w39 _] -> _
    tunnel: w12 -> [w28 _]
    tunnel: w1 -> [w27 _]
    frame No Error {
      n13 = case shown="True" w51 {
        tunnel: w48 -> [_ w121]
        tunnel: w54 -> [w116 w120]
        tunnel: [w117 w119] -> w50
        tunnel: w53 -> [w117 _]
        tunnel: [w116 w118] -> w42
        frame False {
        }
        frame True {
          n14 = property class="Project"(reference=w121, error in=w120) -> (error out=w118:errorcluster, "My Computer"=w119:refnum<vi>)  [unwired: 1 out]
        }
      }
      n15 = call <vilib>:"Has LLB Extension.vi"("path"=w35) -> ("path to VI library?"=w34:bool)
      n16 = Format Into String(format string="%s.lvclass", w30) -> (resulting string=w45:string)  [unwired: 2 in, 1 out]
      n17 = Search and Replace String(replace all?=TRUE ("replace all? (F)"), input string=w27, search string="EmptyClass", replace string=w30) -> (result string=w29:string)  [unwired: 4 in, 3 out]
      n18 = case shown="False" w34 {
        tunnel: [w60 w69] -> w44
        tunnel: w35 -> [w57 w68]
        tunnel: w45 -> [w61 w70]
        tunnel: [w59 w71] -> w43
        tunnel: w42 -> [w58 w66]
        tunnel: w30 -> [_ _]
        tunnel: w28 -> [_ w64]
        tunnel: w29 -> [w55 w63]
        frame False {
          n19 = call <vilib>:"Create Directory Recursive.vi"("directory"=w57) -> ("directory copy"=w56:path)  [unwired: 4 in, 2 out]
          n20 = Build Path(base path=w56, name or relative path=w61) -> (appended path=w60:path)
          n21 = Write to Text File(file (use dialog)=w60, text=w55, error in=w58) -> (error out=w59:errorcluster)  [unwired: 1 in, 2 out]
        }
        frame True {
          n22 = Strip Path(path=w68) -> (stripped path=w67:path)  [unwired: 1 out]
          n23 = call <vilib>:"Create Directory Recursive.vi"("error in (no error)"=w66, "directory"=w67) -> ("error out"=w65:errorcluster, "directory copy"=w62:path)  [unwired: 3 in, 1 out]
          n24 = case shown="False" w64 {
            tunnel: [w73 w93] -> w71
            tunnel: w70 -> [w79 w91]
            tunnel: [w77 w90] -> w69
            tunnel: w68 -> [w80 w89]
            tunnel: w65 -> [w83 w88]
            tunnel: w63 -> [w86 _]
            tunnel: w62 -> [w85 _]
            frame False {
              n25 = Build Path(base path=w85, name or relative path=w79) -> (appended path=w72:path)
              n26 = Write to Text File(file (use dialog)=w72, text=w86, error in=w83) -> (error out=w84:errorcluster)  [unwired: 1 in, 2 out]
              n27 = Build Path(base path=w80, name or relative path=w79) -> (appended path=w77:path)
              n28 = call <vilib>:"New VI Library.vi"("error in (no error)"=w84, "VI library path in"=w80) -> ("error out"=w82:errorcluster)  [unwired: 8 in, 1 out]
              n29 = call "GDSLvClass_OpenClass.vi"("ClassToOpen"=w72, "error in (no error)"=w82) -> ("LVClass.Open"=w81:refnum<vi>, "error out"=w78:errorcluster)  [unwired: 16 in]
              n30 = invoke class="LVClassLibrary" method="Save"(reference=w81, error in=w78, "Path"=w77) -> (reference out=w75:refnum<vi>, error out=w76:errorcluster)  [unwired: 1 in, 2 out]
              n31 = Close Reference(reference=w75, error in (no error)=w76) -> (error out=w74:errorcluster)
              n32 = Delete(path (use dialog)=w72, error in=w74) -> (error out=w73:errorcluster)  [unwired: 3 in, 2 out]
            }
            frame True {
              w87 = "RSRC\r\n\u0000\u0003LVARLBVW\u0000\u0000=Ì\u0000\u0000\u0001ó\u0000\u0000\u0000 \u0000\u0000=¬\u0000\u0000\u0000\u0004\u0000\u0000\u0000\u0000\u0000\u0000\u0000\u0004\u0000\u0000\u0000\u0000\u0000\u0000\u0000\u0004\u0000\u0000\u0000\u0000\u0000\u0000\u0000\u0004\u0000\u0000\u0000\u0000\u0000\u0000\u0000\u0000\u0000\u0000\u0000\u0000\u0000\u0000\u0000\u0000\"\u0000\u0000\u0000>\u0000\u0000\u0003æ\u0000\u0000\u0018>\u0000\u0000\u0018\"\u0000\u0000\u0000\u0000\u0000\u0000\u001fÿÿø\u0000\u0000\u0000\u0000\u0000\u0000\u0000\u0000\u0000@\u0000\u0000\u0004\u0004\u0000\u0000\u0000à\u0001À\u0001\u0002 \u0002\u0005Ð\nJ\u0005Ð\u0002\b\u0005Ð\u0001\u0010\u0002 \u0000à\u0001À\u0000\u0000\u0000\u0000\u0007þ\u0001à\u0002B\u001a\u0010\u0006¢\u0002\u0010\u0003&\u001a\u0010\u0006*\u0003ð\u0002\u0012\u001bð\u0007þ\u0003ð\u0002ª\u001bð\u0000\u0000\u0001à\u0000\u0000\u0000\u0000\u0000\u0000\u0000\u0000\u0000\u0000\u0000\u0000\u0000\u0000\u0000\u0000\u0000\u0000\u0000\u0000\"\u0000\u0000\u0000>\u0000\u0000\u0003æ\u0000\u0000\u0018>\u0000\u0000\u0018\"\u0000\u0000\u0000\u0000\u0000\u0000\u001fÿÿø\u0000\u0000\u0000\u0000\u0000\u0000\u0000\u0000\u0006\u0000\u001fð\u0005\u0010\u0010\u0004`\u0012\u0004\u0014P\u0005Ä\u0011\u0010\u0004\u0014P\u0004`\u0012\u0005\u0010\u0010\u0006\u0000\u001fð\u0000\u0000\u0000\u0000\u0007ü\u0018\u0000\u0004\u0004\u0016\u0000\u0005\u0011\u0005\u0010`\u0006L\u0016\u0010\u0006L\u0010`\u00044\u0011\u00044\u0016\u0000\u0007ü\u0018\u0000\u0000\u0000\u0000\u0000\u0000\u0000\u0000\u0000\u0000\u0000\u0002\u0000\u0000\u0000\u0000\u0000\u0000\u0000\u0000\u0000\u0000\u0000\u0000\u0000\u0000\u0000\u0000\u0000\u0000\u0000\u0000\u0000\u0000\u0000\u0000\u0000\u0000\u0000\u0000\u0000\u0000\u0000\u0000\u0000\u0000\u0000\u0000\u0000\u0000ð\u0000ð\u0000\u0000\u0000\u0000\u0000\u0000\u0000\u0000\u0000\u0000\u0000\u0000\u0000ÿÿð\u0000\u0000\u0000\u0000\u0000\u0000\u0000\u0000\u0000\u0000\u0000ÿÿð\u000fð\u0000\u0000\u0000\u0000\u0000\u0000\u0000\u0000\u0000\u000fð\u0000\u0000ÿÿð\u0000\u0000\u0000\u0000\u0000\u0000\u0000\u0000\u0000\u000fð\u0000\u0000ð\u0000ð\u0000\u0000\u0000\u0000\u0000\u0000\u0000\u0000\u0000\u0000\u0000\u0000\u0000\u0000\u0000\u0000\u0000\u0000\u0000\u0000\u0000\u0000\u0000\u0000\u0000\u000fÿÿÿÿÿÿÿÿÿÿÿÿð\u0000\u0000\u0000\u0000\u0000\u0000\u0000\u0000\u0000\u0000\u0000\u0000\u0000\u0000\u0000\u0000\u0000\u0000\u0000\u0000\u0000\u0000\u0000\u0000\u0000\u0000\u0000\u0000\u0000\u0000\u0000\u0000\u0000\u0000\u0000\u0000\u0000\u000f\u0000\u0000\u0000\u0000\u0000\u0000\u0000\u0000\u0000\u0000\u0000\u0000\u0000\u000f\u0000\u0000\u0000\u000f\u0000\u0000\u0000\u0000\u0000\u0000\u0000\u0000\u0000\u0000\u0000\u0000\u0000ÿð\u0000\u0000\u0000\u0000\u0000\u000fÿ\u0000\u0000\u0000\u0000\u0000\u0000\u000f0Ï\u0000\u0000\u0000\u0000\u0000üÌð\u0000\u0000\u0000\u0000\u0000ð<Íð\u0000\u0000\u0000\u000fÈøß\u0000\u0000\u0000\u0000ððÃÍðð\u0000\u0000\u000fÏ..."  # EmptyClass.lvclass in LLB
              n33 = Write to Text File(file (use dialog)=w89, text=w87, error in=w88) -> (error out=w94:errorcluster)  [unwired: 1 in, 2 out]
              n34 = Build Path(base path=w89, name or relative path="EmptyClass.lvclass") -> (appended path=w92:path)
              n35 = call <vilib>:"Librarian Rename.vi"("error in (no error)"=w94, "new name"=w91, "path"=w92) -> ("error out"=w93:errorcluster, "new path"=w90:path)  [unwired: 7 in]
            }
          }
        }
      }
      n36 = invoke class="ProjectItem" method="AddItem"(reference=w50, error in=w43, "Name"=w45, "Path"=w44, "Type"="LVClass") -> (reference out=w46:refnum<vi>, error out=w41:errorcluster, "AddItem"=w47:refnum<vi>)  [unwired: 1 in, 3 out]
      n37 = Unbundle(w41) -> ("status"=w33:bool)  [unwired: 2 out]
      n38 = Or(x=w34, y=w33) -> ()  [unwired: 1 out]
      n39 = case shown="False" w33 {
        tunnel: w47 -> [w100 w104]
        tunnel: [w96 w109] -> w40
        tunnel: w43 -> [w99 w103]
        tunnel: [w98 w106] -> w37
        tunnel: w48 -> [_ w111]
        tunnel: w44 -> [_ w101]
        frame False {
          w97 = refnum<vi> refnum  # LVClassLibrary
          n40 = To More Specific Class(target class=w97, reference=w100, error in=w99) -> (specific class reference=w96:refnum<vi>, error out=w98:errorcluster)
        }
        frame True {
          # "Is it a Autopopulating folder?"
          n41 = Close Reference(reference=w104, error in (no error)=w103) -> (error out=w102:errorcluster)
          n42 = property class="Project"(reference=w111, error in=w102) -> (error out=w108:errorcluster, "App Ref"=w110:refnum<vi>)  [unwired: 1 out]
          n43 = invoke class="App" method="LVClass.Open"(reference=w110, error in=w108, "Path"=w101) -> (reference out=w105:refnum<vi>, error out=w107:errorcluster, "LVClass.Open"=w109:refnum<vi>)  [unwired: 1 in, 1 out]
          n44 = Close Reference(reference=w105, error in (no error)=w107) -> (error out=w106:errorcluster)
        }
      }
      n45 = property class="LVClassLibrary"(reference=w40) -> (reference out=w38:refnum<vi>, "Type String"=w39:string)  [unwired: 1 in, 1 out]
      n46 = case shown="True" w51 {
        tunnel: w37 -> [w112 w115]
        tunnel: [w112 w114] -> w36
        tunnel: w46 -> [_ w113]
        frame False {
        }
        frame True {
          n47 = Close Reference(reference=w113, error in (no error)=w115) -> (error out=w114:errorcluster)
        }
      }
    }
    frame Error {
    }
  }
  "Project Refnum Out" <- w21
  "error out" <- w25
  "Class Refnum Out" <- w17
  "ClassPathOut" <- w18
